vi "GUI.vi"() -> ()   [LabVIEW 2021]
uses:
  controls/UI Data.ctl
  controls/Data.ctl
  <vilib>/Utility/miscctls.llb/LVTextColorsTypeDef.ctl
  <vilib>/Instr/_visa.llb/VISA Flush IO Buffer Mask.ctl
  <vilib>/Instr/_visa.llb/VISA Set IO Buffer Mask.ctl
  2235c835-d075-488e-97a8-ff40b99ec252.vi
  7fd0a03c-babe-4245-89f2-70f68a4e02e0.vi
  1471845a-d6a4-4e2a-9e95-cd8e6e7553b6.vi
  855ea0af-0154-4148-8bb7-d6a0285b6b06.vi
  67ce05d8-96ad-4a67-b405-b48edab3017d.vi
  0a54dc2d-becf-406e-8766-49dcf30bcf8a.vi
  20f714a1-d882-48df-be09-57c36569b2f2.vi
  ebcdb7a2-2a2c-4ba1-9570-780fec90ea4c.vi
  d7b92f73-f523-4b2b-853d-7ace1ccfb4c3.vi
  5e66b44c-e304-46e7-babf-65c984714624.vi
  3f0796be-9eb5-410d-95a1-f686e7479b0e.vi
  a6c2df6f-6ad4-4eb4-a9bc-2f05b466e969.vi
  535851f3-05c5-415e-8a07-50860e4f08cf.vi
  3643a199-7bcb-4f24-a83d-5ca93d957abf.vi
  187f9bc3-0ed3-4701-b56c-3ff7ee860393.vi
  eb7b7dfd-645e-46e6-868f-ba0f7f713db4.vi
  <vilib>/ULx/Write.llb/ULx Write (Digital Bool 1Line 1Point).vi
  <vilib>/Instr/_visa.llb/VISA Configure Serial Port (Instr).vi
  <vilib>/ULx/Create Channel.llb/ULx Create Channel (DO-Digital Output).vi
  styles/colors.vi
  <vilib>/ULx/ULx_LV.dll
  <vilib>/NI/Progress Bar/Progress Bar.lvlib
  <vilib>/zip/NI_Unzip.lvlib
panel:
  in  "Stop button":bool
  in  "Run button":bool
  out "Status":string
  in  "Settings button":bool
  out "Console":string
  in  "Serial communication\n settings":T1={"COM"="", "baud rate"=115200, "data bits"=8, "parity"=enum."None", "stop bits"=10, "flow control"=enum."None", "delay"=50, "I/O channel"="", "Board IP"=""} {"stop bits" items=["1.0"=10, "1.5"=15, "2.0"=20]; "baud rate" max=921600; "data bits" max=16}
  in  "Paths":bool
  in  "Save button":bool
  out "version:":string
  in  "Path: 4.9.12.XXXX":path=path "C:/Users/ken_X/Documents/LabVIEW projects/Project-A/outset-medical/4.9.12.6034"
  in  "Path: Android OS":path=path "C:/Users/ken_X/Documents/LabVIEW projects/Project-A/outset-medical/Android OS"
  # "Serial communication\n settings"
  # "I/O Channel"
  # "Board IP"
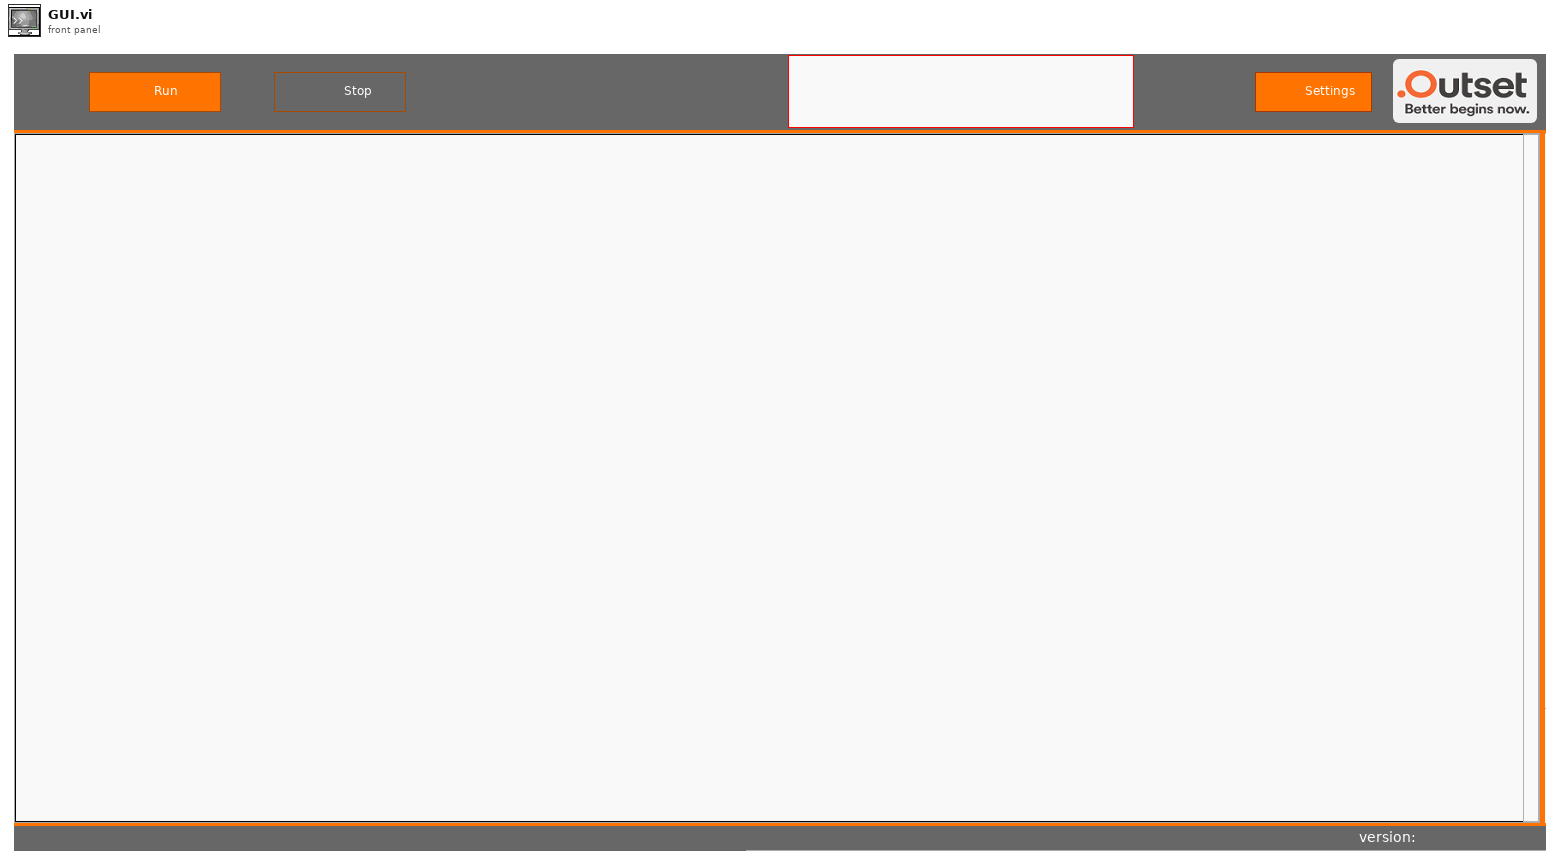
[diagram p1: front panel]
types:
  T1 = cluster{"COM":refnum<visa-resource-name>, "baud rate":u32, "data bits":u8, "parity":enum16{"None", "Odd", "Even", "Mark", "Space"}, "stop bits":u16, "flow control":enum16{"None", "XON/XOFF", "RTS/CTS", "DTR/DSR"}, "delay":u16, "I/O channel":refnum<k21>, "Board IP":string}
  T2 = typedef "Data.ctl" = cluster{"Console":refnum<vi>, "COM":refnum<visa-resource-name>, "Delay":u32, "IO task":refnum<k24>, "Python session":refnum<k35>, "Script path":path, "Media Url":string, "Media version":i32, "Attempts left":i32, "Version path":path, "Android path":path, "Python 2.7":path, "My temp":path, "Board IP":string, "ID Part":string, "Error":string, "Pass?":string}
  T3 = enum8{"Enabled", "Disabled", "Disabled and Grayed Out"}
  T4 = typedef "UI Data.ctl" = cluster{"settings splitter":refnum<vi>, "footer splitter":refnum<vi>, "Serial communication\n settings":refnum<vi>, "Path: Android OS":refnum<vi>, "Path: 4.9.12.XXXX":refnum<vi>}
  T5 = cluster{"primary color":u32, "secondary color":u32, "accent color":u32, "background color":u32, "accent s color":u32}
  T6 = cluster{"accent s color":u32, "accent s color":u32}
  T7 = cluster{"accent s color":u32, "accent color":u32}
  T8 = cluster{"primary color":u32, "primary color":u32}
  T9 = typedef "LVTextColorsTypeDef.ctl" = cluster{"Text Color":u32, "Background Color":u32}
  T10 = enum16{"open", "replace", "create", "open or create", "replace or create", "replace or create with confirmation"}
  T11 = cluster{"Android":path, "Version":path, "Labview Script":path, "Python 2.7":path, "My temp":path}
  T12 = typedef "VISA Set IO Buffer Mask.ctl" = u16
  T13 = typedef "VISA Flush IO Buffer Mask.ctl" = u16
  T14 = cluster{"secondary color":u32, "secondary color":u32}
  T15 = cluster{"Value":path, "Value":path, path, path, path}
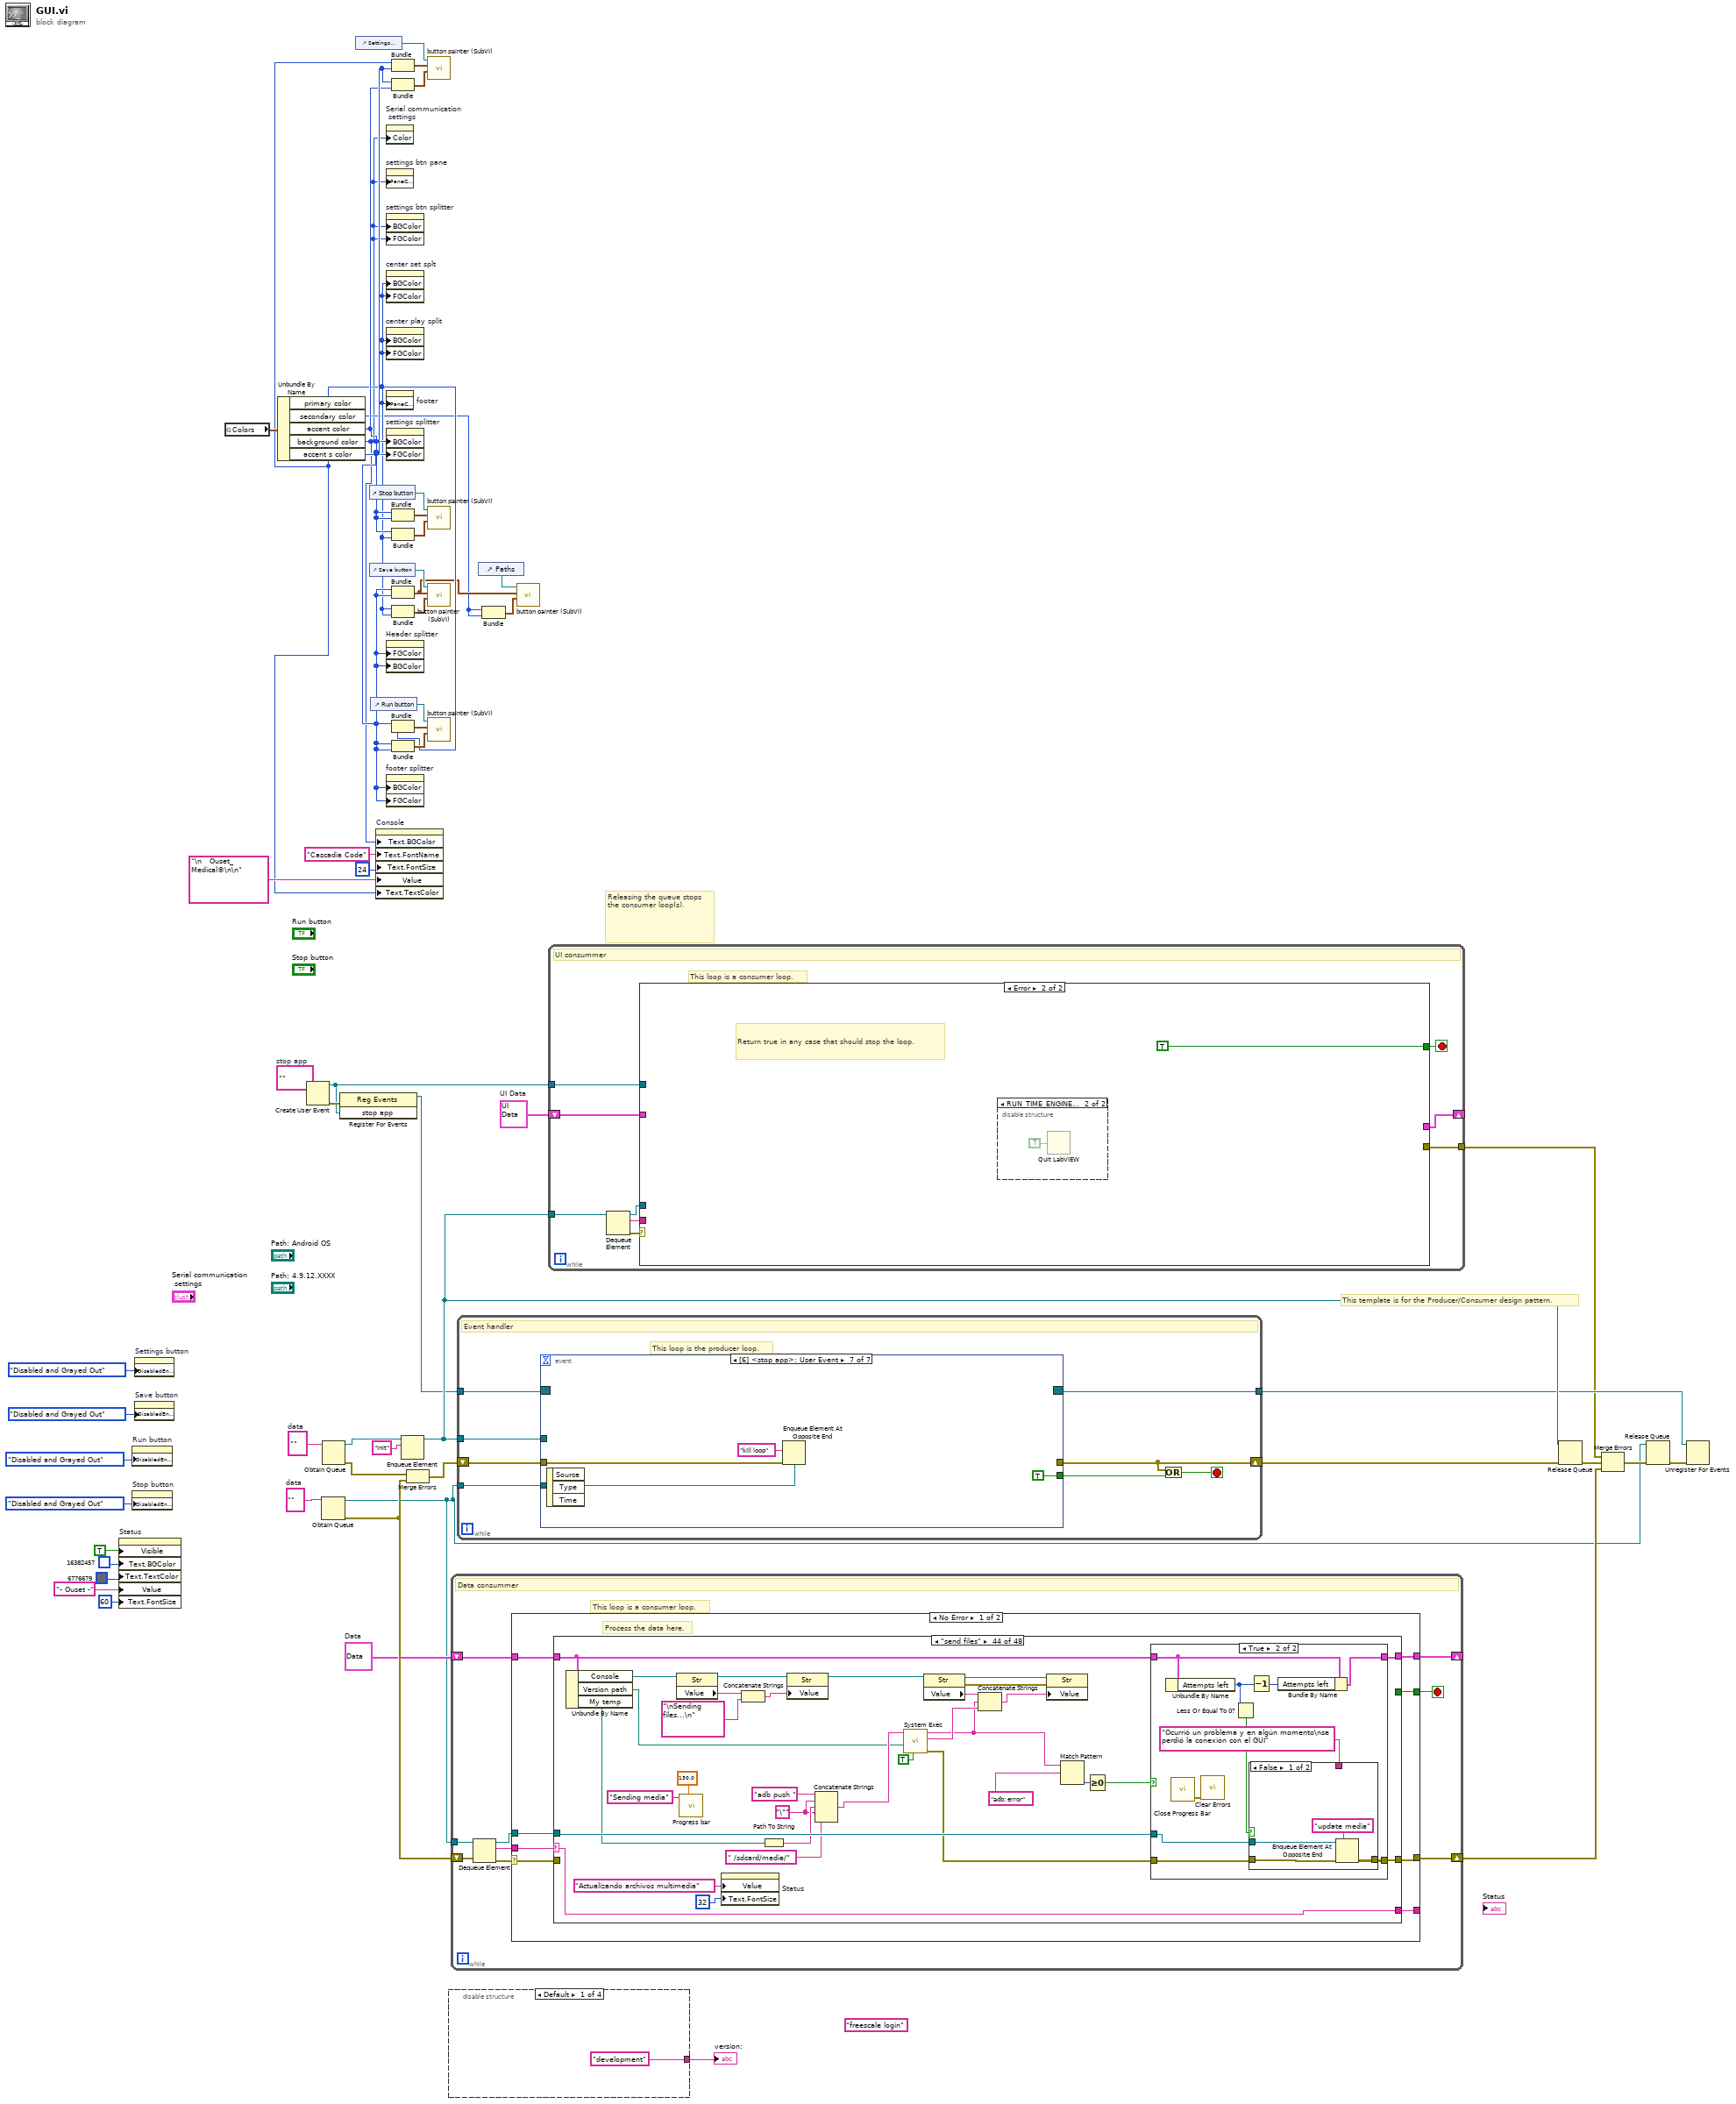
[diagram p0: block diagram]
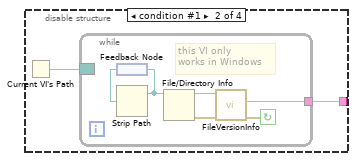
[diagram p2: hidden frame]
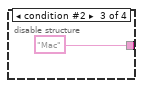
[diagram p3: hidden frame]
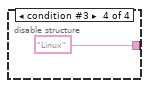
[diagram p4: hidden frame]
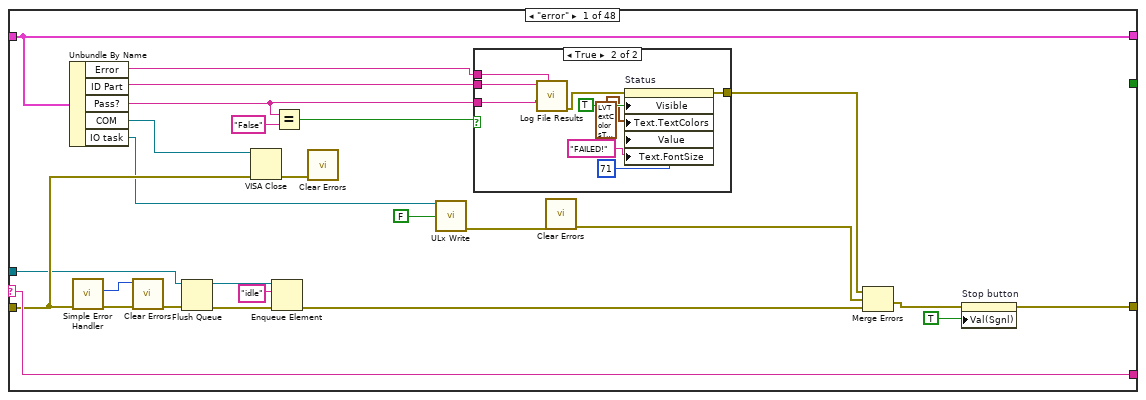
[diagram p5: hidden frame]
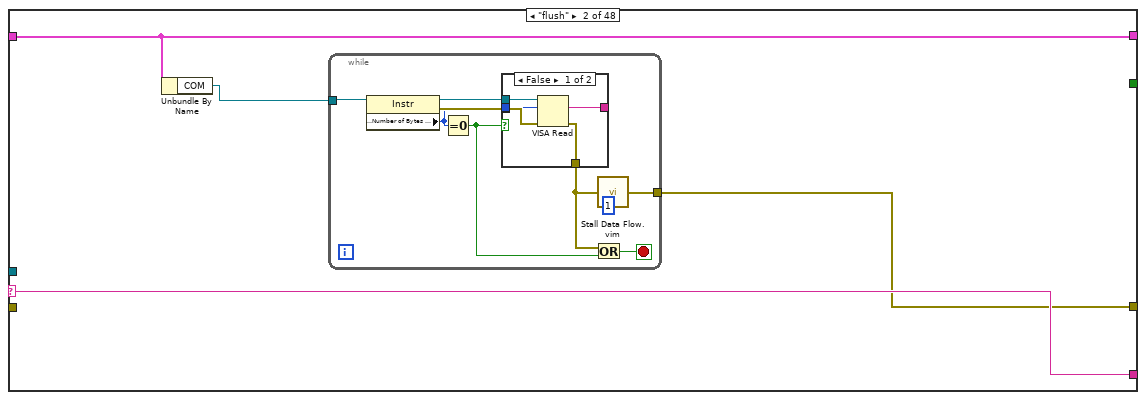
[diagram p7: hidden frame]
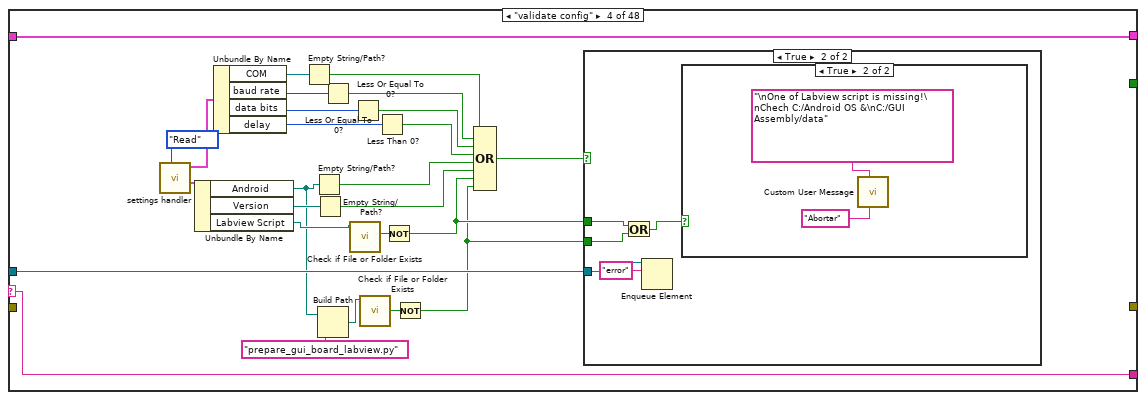
[diagram p10: hidden frame]
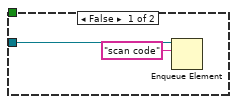
[diagram p11: hidden frame]
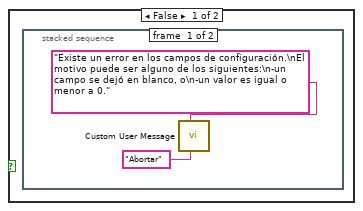
[diagram p12: hidden frame]
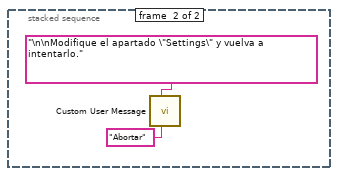
[diagram p13: hidden frame]
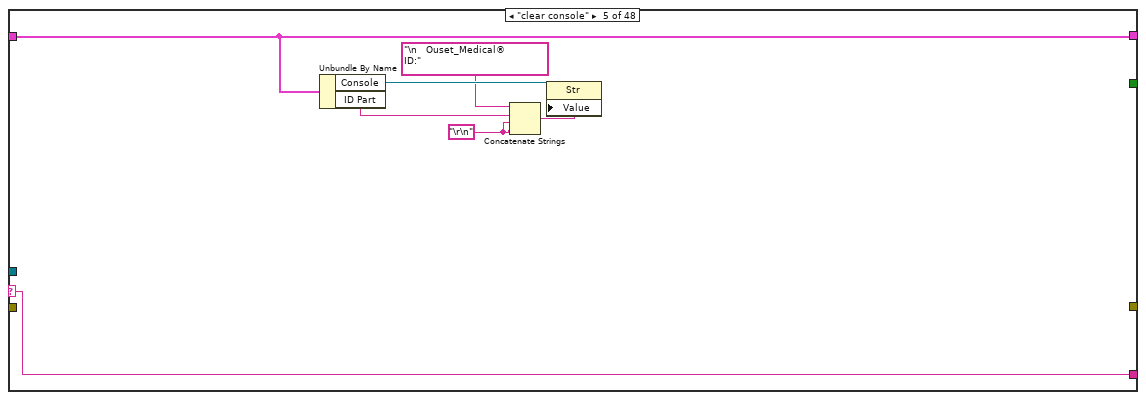
[diagram p14: hidden frame]
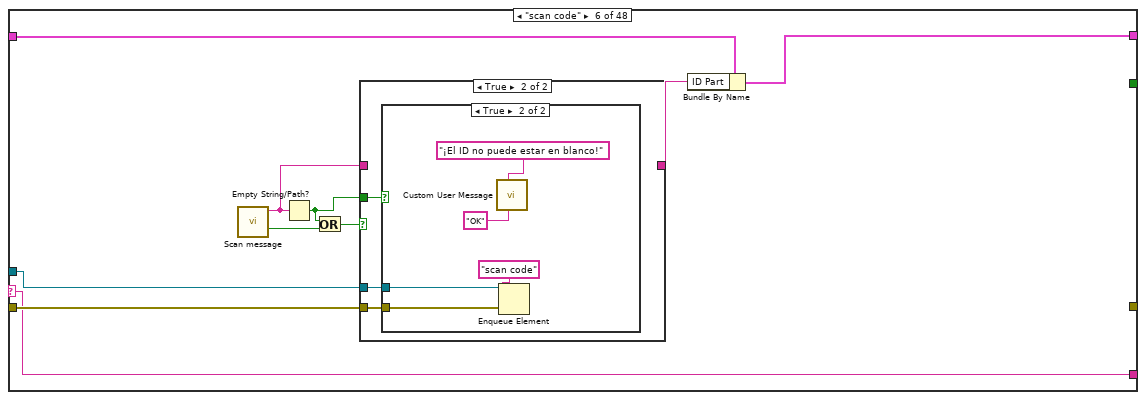
[diagram p15: hidden frame]
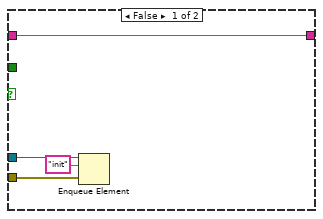
[diagram p16: hidden frame]
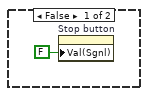
[diagram p17: hidden frame]
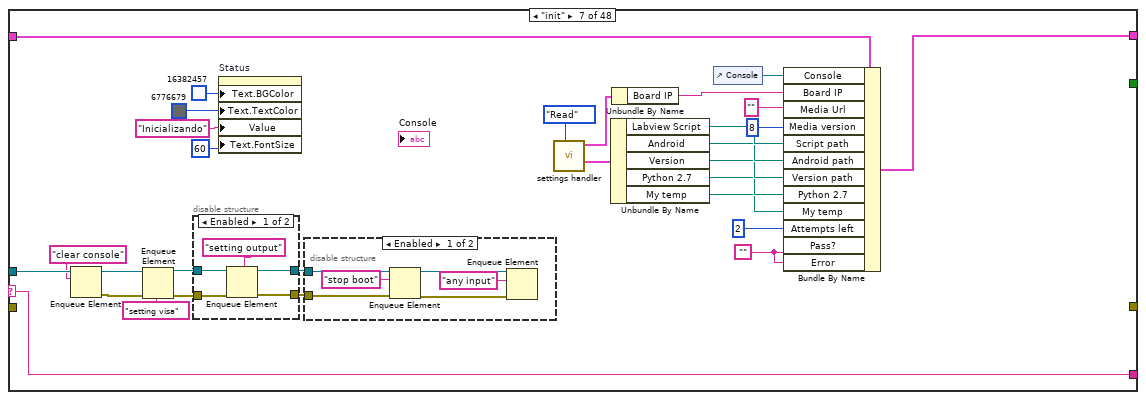
[diagram p18: hidden frame]
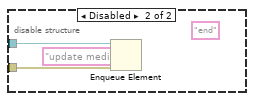
[diagram p20: hidden frame]
diagram:
  (unwired) "freescale login"
  w15 = T2 {"Console"=refnum, "COM"="", "Delay"=50, "IO task"=refnum, "Python session"=refnum, "Script path"=path "C:/Users/ken_X/Documents/LabVIEW projects/Project-A/Update_Media_bi.py", "Media Url"="", "Media version"=0, "Attempts left"=3, "Version path"=path "C:/Users/ken_X/Documents/LabVIEW projects/Project-A/Update_Media_bi.py", "Android path"=path "C:/Users/ken_X/Documents/LabVIEW projects/Project-A/Update_Media_bi.py", "Python 2.7"=path "C:/Users/ken_X/Documents/LabVIEW projects/Project-A/Update_Media_bi.py", "My temp"=path "C:/Users/ken_X/Documents/LabVIEW projects/Project-A/Update_Media_bi.py", "Board IP"="", "ID Part"="", "Error"="", "Pass?"=""}  # Data
  w33 = ""  # data
  w46 = ""  # stop app
  w50 = T4 {"settings splitter"=refnum, "footer splitter"=refnum, "Serial communication\n settings"=refnum, "Path: Android OS"=refnum, "Path: 4.9.12.XXXX"=refnum}  # UI Data
  w47 = ""  # data
  # "Releasing the queue stops the consumer loop(s)."
  # "This template is for the Producer/Consumer design pattern."
  n1 = property on="Status" class="Str"("Visible"=TRUE, "Text.BGColor"=u32 16382457 ("background color"), "Text.TextColor"=u32 6776679 ("primary color"), "Value"="- Ouset -" ("Status"), "Text.FontSize"=u32 60 ("Text.Font:Size")) -> ()  [unwired: 2 in, 2 out]
  n2 = property on="Run button" class="Bool (strict)"("DisabledEnum"=T3."Disabled and Grayed Out" ("Disabled")) -> ()  [unwired: 2 in, 2 out]
  n3 = property on="Stop button" class="Bool (strict)"("DisabledEnum"=T3."Disabled and Grayed Out" ("Disabled")) -> ()  [unwired: 2 in, 2 out]
  n4 = property on="Settings button" class="Bool (strict)"("DisabledEnum"=T3."Disabled and Grayed Out" ("Disabled")) -> ()  [unwired: 2 in, 2 out]
  n5 = property on="Save button" class="Bool (strict)"("DisabledEnum"=T3."Disabled and Grayed Out" ("Disabled")) -> ()  [unwired: 2 in, 2 out]
  n6 = global read "colors.vi" "Colors"() -> (w55:T5)
  n7 = Unbundle By Name(w55) -> ("primary color"=w22:u32, "secondary color"=w18:u32, "accent color"=w23:u32, "background color"=w16:u32, "accent s color"=w24:u32)
  n8 = Create User Event(user event datatype=w46) -> (user event=w44:refnum<user-event>, error out=w45:errorcluster)  [unwired: 1 in]
  n9 = Obtain Queue(element data type=w33) -> (queue out=w5:refnum<queue>, error out=w30:errorcluster)  [unwired: 4 in, 1 out]
  n10 = Obtain Queue(element data type=w47) -> (queue out=w53:refnum<queue>, error out=w32:errorcluster)  [unwired: 4 in, 1 out]
  n11 = register-events(error in=w45, w44) -> (reference out=w14:refnum<event-registration>)  [unwired: 1 in, 1 out]
  n12 = control-ref of="Settings button"() -> (w38:refnum<vi>)
  n13 = control-ref of="Stop button"() -> (w36:refnum<vi>)
  n14 = control-ref of="Save button"() -> (w37:refnum<vi>)
  n15 = control-ref of="Run button"() -> (w43:refnum<vi>)
  n16 = property on="Console" class="Str"("Text.BGColor"=w16, "Text.FontName"="Cascadia Code" ("Text.Font:Name"), "Text.FontSize"=u32 24 ("Text.Font:Size"), "Value"="\n   Ouset_Medical®\n\n" ("Console"), "Text.TextColor"=w24) -> ()  [unwired: 2 in, 2 out]
  n17 = property on="Serial communication\n settings" class="Clust (strict)"("Color"=w16) -> ()  [unwired: 2 in, 2 out]
  n18 = property on="settings btn pane" class="Pane"("PaneColor"=w16) -> ()  [unwired: 2 in, 2 out]
  n19 = property on="settings btn splitter" class="Splitter"("BGColor"=w16, "FGColor"=w16) -> ()  [unwired: 2 in, 2 out]
  n20 = property on="center set splt" class="Splitter"("BGColor"=w22, "FGColor"=w22) -> ()  [unwired: 2 in, 2 out]
  n21 = property on="center play split" class="Splitter"("BGColor"=w22, "FGColor"=w22) -> ()  [unwired: 2 in, 2 out]
  n22 = property on="footer" class="Pane"("PaneColor"=w22) -> ()  [unwired: 2 in, 2 out]
  n23 = property on="settings splitter" class="Splitter"("BGColor"=w23, "FGColor"=w23) -> ()  [unwired: 2 in, 2 out]
  n24 = property on="Header splitter" class="Splitter"("FGColor"=w23, "BGColor"=w23) -> ()  [unwired: 2 in, 2 out]
  n25 = property on="footer splitter" class="Splitter"("BGColor"=w23, "FGColor"=w23) -> ()  [unwired: 2 in, 2 out]
  n26 = Bundle("accent s color"=w24, "accent s color"=w24) -> (w40:T6)  [unwired: 1 in]
  n27 = Bundle("accent s color"=w24, "accent color"=w23) -> (w39:T7)  [unwired: 1 in]
  n28 = Bundle("accent color"=w23, "accent color"=w23) -> (w34:cluster{"accent color":u32, "accent color":u32})  [unwired: 1 in]
  n29 = Bundle("accent color"=w23, "primary color"=w22) -> (w35:cluster{"accent color":u32, "primary color":u32})  [unwired: 1 in]
  n30 = Bundle("accent color"=w23, "accent color"=w23) -> (w20:cluster{"accent color":u32, "accent color":u32})  [unwired: 1 in]
  n31 = Bundle("primary color"=w22, "primary color"=w22) -> (w19:T8)  [unwired: 1 in]
  n32 = Bundle("accent color"=w23, "primary color"=w22) -> (w41:cluster{"accent color":u32, "primary color":u32})  [unwired: 1 in]
  n33 = Bundle("accent color"=w23, "accent color"=w23) -> (w42:cluster{"accent color":u32, "accent color":u32})  [unwired: 1 in]
  n34 = Enqueue Element(queue=w53, element="init") -> (queue out=w52:refnum<queue>)  [unwired: 2 in, 2 out]
  n35 = Merge Errors(w32, w30) -> (w31:errorcluster)
  n36 = call "button painter (SubVI).vi"("Off state"=w39, "On state"=w40, "Button ref in"=w38) -> ()  [unwired: 9 in]
  n37 = call "button painter (SubVI).vi"("Off state"=w35, "On state"=w34, "Button ref in"=w36) -> ()  [unwired: 9 in]
  n38 = call "button painter (SubVI).vi"("Off state"=w19, "On state"=w20, "Button ref in"=w37) -> ()  [unwired: 9 in]
  n39 = call "button painter (SubVI).vi"("Off state"=w42, "On state"=w41, "Button ref in"=w43) -> ()  [unwired: 9 in]
  n40 = disable-structure "Conditional Disable Structure" shown="Default" {
    disable-tunnel: ["development" w57 "Mac" "Linux"] -> w13
    frame condition #0 (active) {
    }
    frame condition #1 {
      n41 = Current VI's Path() -> (path=w58:path)
      n42 = while {
        border: w58 -> [_]
        tunnel: [w59] -> w57
        stop <- w63 continue-if-true
        # "this VI only \nworks in Windows"
        n43 = feedback #1() -> (w62:path)
        n44 = Strip Path(path=w62) -> (stripped path=w61:path)  [unwired: 1 out]
        n45 = feedback-in #1(w61) -> ()
        n46 = File/Directory Info(path=w61) -> (path out=w60:path, error out=w64:errorcluster)  [unwired: 1 in, 5 out]
        n47 = call <vilib>:"FileVersionInfo.vi"("error in (no error)"=w64, "Application Path in"=w60) -> ("error out"=w63:errorcluster, "File Version Info"=w59:string)  [unwired: 6 in, 2 out]
      }
    }
    frame condition #2 {
    }
    frame condition #3 {
    }
  }
  "version:" <- w13
  n48 = while {
    tunnel: w5 -> [w75]
    shift-right: [w69] -> _
    shift-left: w15 -> [w70]
    shift-right: [w67] -> w8
    shift-left: w30 -> [w71]
    stop <- w68 stop-if-true
    # "This loop is a consumer loop."
    # "Data consummer"
    n49 = Dequeue Element(queue=w75, error in (no error)=w71) -> (queue out=w72:refnum<queue>, element=w73:string, error out=w74:errorcluster)  [unwired: 1 in, 1 out]
    n50 = case shown="No Error" w74 {
      selector: w74 -> [w78 w1835]
      tunnel: w73 -> [w83 _]
      tunnel: w72 -> [w82 w1843]
      tunnel: w70 -> [w81 w1842]
      tunnel: [w80 w1842] -> w69
      tunnel: [w79 "ERROR"] -> _
      tunnel: [w77 w1838] -> w67
      tunnel: [w76 _] -> w68
      frame No Error {
        # "Process the data here."
        n51 = case shown="\"send files\"" w83 {
          selector: w83 -> [w108 w121 w138 w148 w183 w187 w234 w264 w315 w363 w399 w441 w507 w541 w574 w638 w668 w707 w738 w801 w862 w903 w929 w989 w1032 w1054 w1091 w1126 w1179 w1217 w1268 w1291 w1345 w1363 w1385 w1425 w1469 w1505 w1530 w1553 w1591 w1629 w1662 w1708 w1759 w1779 w1788 w1804]
          tunnel: w82 -> [w97 _ _ w149 _ w194 w238 _ _ w364 w400 w444 w508 w545 w577 _ w669 w706 w739 w804 w852 _ w936 w990 _ w1056 w1093 w1128 w1180 w1219 _ w1293 w1347 _ w1380 w1418 w1463 w1507 w1527 w1556 w1594 w1632 w1655 w1710 w1761 _ _ w1800]
          tunnel: w81 -> [w86 w122 w139 w165 w185 w191 w237 w256 w321 w361 w413 w436 w490 w542 w569 w637 w666 w709 w736 w800 w836 w917 w922 w987 w1035 w1044 w1086 w1109 w1172 w1203 w1258 w1278 w1321 w1359 w1376 w1417 w1452 w1503 w1532 w1541 w1579 w1617 w1666 w1685 w1752 w1777 w1789 w1799]
          tunnel: [w86 w122 w139 w165 w185 w190 w235 w270 w325 w361 w413 w435 w489 w542 w570 w637 w666 w709 w736 w800 w835 w917 w921 w987 w1034 w1043 w1085 w1108 w1171 w1202 w1258 w1277 w1321 w1359 w1374 w1417 w1450 w1503 w1532 w1540 w1578 w1616 w1666 w1684 w1752 w1777 w1789 w1799] -> w80
          tunnel: [w108 w121 w138 w148 w183 w187 w234 w264 w315 w363 w399 w441 w507 w541 w574 w638 w668 w707 w738 w801 w862 w903 w929 w989 w1032 w1054 w1091 w1126 w1179 w1217 w1268 w1291 w1345 w1363 w1385 w1425 w1469 w1505 w1530 w1553 w1591 w1629 w1662 w1708 w1759 w1779 w1788 w1804] -> w79
          tunnel: w78 -> [w100 _ _ _ _ w195 _ _ w337 _ w404 _ _ _ _ _ _ _ _ w810 w850 _ w934 _ _ w1051 _ w1124 w1177 w1212 _ _ _ w1361 w1382 w1421 _ w1506 w1529 _ _ _ w1654 _ _ _ _ _]
          tunnel: [w103 w119 _ _ _ _ _ w262 w322 w358 w401 w437 w495 w540 w572 w629 w663 w704 w733 w803 w848 _ w933 w984 w1031 w1052 w1092 w1125 w1178 w1213 w1259 w1289 w1333 w1360 w1379 w1419 w1464 w1504 w1528 w1551 w1589 w1627 w1664 w1706 w1757 w1772 _ w1801] -> w77
          tunnel: [_ _ _ _ _ _ _ _ _ _ _ _ _ _ _ _ _ _ _ _ _ _ _ _ _ _ _ _ _ _ _ _ _ _ _ _ _ _ _ _ _ _ _ _ _ _ TRUE _] -> w76
          frame "error" {
            n52 = Unbundle By Name(w86) -> ("Error"=w92:string, "ID Part"=w93:string, "Pass?"=w94:string, "COM"=w105:refnum<visa-resource-name>, "IO task"=w91:refnum<k24>)
            n53 = call <vilib>:"Simple Error Handler.vi"("error in (no error)"=w100) -> ("code out"=w101:i32, "error out"=w98:errorcluster)  [unwired: 4 in, 3 out]
            n54 = call <vilib>:"Clear Errors.vi"("error in (no error)"=w98, "specific error code to clear (0: all)"=w101) -> ("error out"=w99:errorcluster)  [unwired: 4 in, 1 out]
            n55 = Flush Queue(queue=w97, error in (no error)=w99) -> (queue out=w107:refnum<queue>, error out=w106:errorcluster)  [unwired: 1 out]
            n56 = VISA Close(VISA resource name=w105, error in (no error)=w100) -> (error out=w102:errorcluster)
            n57 = Enqueue Element(queue=w107, element="idle", error in (no error)=w106) -> (error out=w88:errorcluster)  [unwired: 1 in, 2 out]
            n58 = Equal?(x=w94, y="False") -> (x = y?=w96:bool)
            n59 = call <vilib>:"Clear Errors.vi"("error in (no error)"=w102) -> ()  [unwired: 5 in, 2 out]
            n60 = call-poly <vilib>:"ULx Write.vi"("task in"=w91, "data"=FALSE) -> ("error out"=w85:errorcluster)  [unwired: 11 in, 2 out]
            n61 = case shown="True" w96 {
              tunnel: w93 -> [_ w118]
              tunnel: w94 -> [_ w117]
              tunnel: w92 -> [_ w116]
              tunnel: [_ w111] -> w89
              frame False {
              }
              frame True {
                n62 = call "Log File Results.vi"("Error"=w116, "Pass?"=w117, "Part Number"=w118) -> ("error out"=w112:errorcluster)  [unwired: 8 in]
                n63 = property on="Status" class="Str"(error in=w112, "Visible"=TRUE, "Text.TextColors"=T9 {"Text Color"=16777225, "Background Color"=16711680} ("Text.Text Colors"), "Value"="FAILED!" ("Status"), "Text.FontSize"=u32 71 ("Text.Font:Size")) -> (error out=w111:errorcluster)  [unwired: 1 in, 1 out]
              }
            }
            n64 = call <vilib>:"Clear Errors.vi"("error in (no error)"=w85) -> ("error out"=w84:errorcluster)  [unwired: 5 in, 1 out]
            n65 = Merge Errors(w89, w84, w88) -> (w87:errorcluster)
            n66 = property on="Stop button" class="Bool (strict)"(error in=w87, "Val(Sgnl)"=TRUE ("Value (Signaling)")) -> (error out=w103:errorcluster)  [unwired: 1 in, 1 out]
          }
          frame "flush" {
            n67 = Unbundle By Name(w122) -> ("COM"=w120:refnum<visa-resource-name>)
            n68 = while {
              tunnel: w120 -> [w131]
              tunnel: [w124] -> w119
              stop <- w129 stop-if-true
              n69 = property class="Instr"(reference=w131) -> (reference out=w130:refnum<visa-resource-name>, error out=w128:errorcluster, "Serial Settings:Number of Bytes at Serial Port"=w126:u32)  [unwired: 1 in]
              n70 = Equal To 0?(x=w126) -> (x = 0?=w127:bool)
              n71 = case shown="False" w127 {
                tunnel: w130 -> [w136 _]
                tunnel: w128 -> [w135 w137]
                tunnel: [w134 w137] -> w125
                tunnel: w126 -> [w133 _]
                tunnel: [w132 _] -> _
                frame False {
                  n72 = VISA Read(VISA resource name=w136, byte count=w133, error in (no error)=w135) -> (read buffer=w132:string, error out=w134:errorcluster)  [unwired: 2 out]
                }
                frame True {
                }
              }
              n73 = Or(x=w125, y=w127) -> (x .or. y?=w129:bool)
              n74 = call "Stall Data Flow.vim"("value in"=w125, "milliseconds to wait"=u32 1) -> ("value out"=w124:errorcluster)  [unwired: 1 out]
            }
          }
          frame "idle", Default {
          }
          frame "validate config" {
            n75 = call "settings handler.vi"("Operation"=enum16{"Open", "Write", "Read", "Close"}."Read") -> ("Paths read"=w163:T11, "Read"=w159:T1)  [unwired: 8 in, 1 out]
            n76 = Unbundle By Name(w163) -> ("Android"=w143:path, "Version"=w162:path, "Labview Script"=w147:path)
            n77 = Unbundle By Name(w159) -> ("COM"=w158:refnum<visa-resource-name>, "baud rate"=w157:u32, "data bits"=w156:u8, "delay"=w155:u16)
            n78 = Empty String/Path?(string/path=w158) -> (empty?=w151:bool)
            n79 = Empty String/Path?(string/path=w143) -> (empty?=w160:bool)
            n80 = Empty String/Path?(string/path=w162) -> (empty?=w161:bool)
            n81 = Build Path(base path=w143, name or relative path="prepare_gui_board_labview.py") -> (appended path=w144:path)
            n82 = Less Or Equal To 0?(x=w157) -> (x <= 0?=w152:bool)
            n83 = call <vilib>:"Check if File or Folder Exists.vi"("path"=w147) -> ("file or folder exists?"=w146:bool)  [unwired: 8 in, 2 out]
            n84 = Less Or Equal To 0?(x=w156) -> (x <= 0?=w153:bool)
            n85 = call <vilib>:"Check if File or Folder Exists.vi"("path"=w144) -> ("file or folder exists?"=w141:bool)  [unwired: 8 in, 2 out]
            n86 = Less Than 0?(x=w155) -> (x < 0?=w154:bool)
            n87 = Not(x=w146) -> (.not. x?=w145:bool)
            n88 = Not(x=w141) -> (.not. x?=w140:bool)
            n89 = Compound Arithmetic op=OR(w151, w152, w153, w154, w160, w161, w145, w140) -> (w150:bool)
            n90 = case shown="True" w150 {
              tunnel: w149 -> [w167 w172]
              tunnel: w145 -> [_ w170]
              tunnel: w140 -> [_ w169]
              frame False {
                n91 = Enqueue Element(queue=w167, element="scan code") -> ()  [unwired: 2 in, 3 out]
              }
              frame True {
                n92 = Or(x=w170, y=w169) -> (x .or. y?=w168:bool)
                n93 = Enqueue Element(queue=w172, element="error") -> ()  [unwired: 2 in, 3 out]
                n94 = case shown="True" w168 {
                  frame False {
                    n95 = stacked-sequence {
                      frame #0 {
                        n96 = call "Custom User Message.vi"("Button text (\"OK\")"="Abortar" ("Button text (\"OK\")"), "MSG"="Existe un error en los campos de configuración.\nEl motivo puede ser alguno de los siguientes:\n-un campo se dejó en blanco, o\n-un valor es igual o menor a 0." ("message")) -> ()  [unwired: 9 in, 1 out]
                      }
                      frame #1 {
                        n97 = call "Custom User Message.vi"("Button text (\"OK\")"="Abortar" ("Button text (\"OK\")"), "MSG"="\n\nModifique el apartado \"Settings\" y vuelva a intentarlo.") -> ()  [unwired: 9 in, 1 out]
                      }
                    }
                  }
                  frame True {
                    n98 = call "Custom User Message.vi"("Button text (\"OK\")"="Abortar" ("Button text (\"OK\")"), "MSG"="\nOne of Labview script is missing!\nChech C:/Android OS &\nC:/GUI Assembly/data" ("message")) -> ()  [unwired: 9 in, 1 out]
                  }
                }
              }
            }
          }
          frame "clear console" {
            w179 = "\r\n"
            n99 = Unbundle By Name(w185) -> ("Console"=w184:refnum<vi>, "ID Part"=w180:string)
            n100 = Concatenate Strings("\n   Ouset_Medical®         ID:" ("Value"), w180, w179, w179) -> (w182:string)
            n101 = property class="Str"(reference=w184, "Value"=w182) -> ()  [unwired: 1 in, 2 out]
          }
          frame "scan code" {
            n102 = call "Scan message.vi"() -> ("Abort?"=w193:bool, "out"=w188:string)  [unwired: 10 in]
            n103 = Empty String/Path?(string/path=w188) -> (empty?=w186:bool)
            n104 = Or(x=w186, y=w193) -> (x .or. y?=w192:bool)
            n105 = case shown="True" w192 {
              tunnel: w195 -> [w199 w200]
              tunnel: w194 -> [w198 w201]
              tunnel: [w196 _] -> w189
              tunnel: w188 -> [w196 _]
              tunnel: w186 -> [_ w202]
              frame False {
                n106 = Enqueue Element(queue=w198, element="init", error in (no error)=w199) -> ()  [unwired: 1 in, 3 out]
              }
              frame True {
                n107 = case shown="True" w202 {
                  tunnel: w201 -> [_ w207]
                  tunnel: w200 -> [_ w206]
                  frame False {
                    n108 = property on="Stop button" class="Bool (strict)"("Val(Sgnl)"=FALSE ("Value (Signaling)")) -> ()  [unwired: 2 in, 2 out]
                  }
                  frame True {
                    n109 = call "Custom User Message.vi"("Button text (\"OK\")"="OK" ("Button text (\"OK\")"), "MSG"="¡El ID no puede estar en blanco!") -> ()  [unwired: 9 in, 1 out]
                    n110 = Enqueue Element(queue=w207, element="scan code", error in (no error)=w206) -> ()  [unwired: 1 in, 3 out]
                  }
                }
              }
            }
            n111 = Bundle By Name(cluster=w191, "ID Part"=w189) -> (w190:T2)
          }
          frame "init" {
            w218 = ""
            n112 = Enqueue Element(queue=w238, element="clear console") -> (queue out=w221:refnum<queue>, error out=w222:errorcluster)  [unwired: 2 in, 1 out]
            n113 = Enqueue Element(queue=w221, element="setting visa", error in (no error)=w222) -> (queue out=w215:refnum<queue>, error out=w216:errorcluster)  [unwired: 1 in, 1 out]
            n114 = disable-structure shown="Enabled" {
              disable-tunnel: w216 -> [w243 w244]
              disable-tunnel: w215 -> [w242 w245]
              disable-tunnel: [w241 w245] -> w214
              disable-tunnel: [w240 w244] -> w213
              frame Enabled {
                n115 = Enqueue Element(queue=w242, element="setting output", error in (no error)=w243) -> (queue out=w241:refnum<queue>, error out=w240:errorcluster)  [unwired: 1 in, 1 out]
              }
              frame Disabled {
              }
            }
            n116 = property on="Status" class="Str"("Text.BGColor"=u32 16382457 ("background color"), "Text.TextColor"=u32 6776679 ("primary color"), "Value"="Inicializando" ("Status"), "Text.FontSize"=u32 60 ("Text.Font:Size")) -> ()  [unwired: 2 in, 2 out]
            n117 = disable-structure shown="Enabled" {
              disable-tunnel: w214 -> [w251 w254]
              disable-tunnel: w213 -> [w247 w252]
              frame Enabled {
                n118 = Enqueue Element(queue=w251, element="stop boot", error in (no error)=w247) -> (queue out=w249:refnum<queue>, error out=w248:errorcluster)  [unwired: 1 in, 1 out]
                n119 = Enqueue Element(queue=w249, element="any input", error in (no error)=w248) -> ()  [unwired: 1 in, 3 out]
              }
              frame Disabled {
                (unwired) "end" ("element")
                n120 = Enqueue Element(queue=w254, element="update media", error in (no error)=w252) -> ()  [unwired: 1 in, 3 out]
              }
            }
            n121 = call "settings handler.vi"("Operation"=enum16{"Open", "Write", "Read", "Close"}."Read") -> ("Paths read"=w229:T11, "Read"=w219:T1)  [unwired: 8 in, 1 out]
            n122 = Unbundle By Name(w229) -> ("Labview Script"=w228:path, "Android"=w226:path, "Version"=w225:path, "Python 2.7"=w224:path, "My temp"=w223:path)
            n123 = Unbundle By Name(w219) -> ("Board IP"=w220:string)
            n124 = control-ref of="Console"() -> (w236:refnum<vi>)
            n125 = Bundle By Name(cluster=w237, "Console"=w236, "Board IP"=w220, "Media Url"="", "Media version"=8, "Script path"=w228, "Android path"=w226, "Version path"=w225, "Python 2.7"=w224, "My temp"=w223, "Attempts left"=2, "Pass?"=w218, "Error"=w218) -> (w235:T2)
          }
          frame "setting visa" {
            n126 = call "settings handler.vi"("Operation"=enum16{"Open", "Write", "Read", "Close"}."Read") -> ("Read"=w275:T1)  [unwired: 8 in, 2 out]
            n127 = Unbundle By Name(w256) -> ("Console"=w261:refnum<vi>)
            n128 = Unbundle By Name(w275) -> ("COM"=w274:refnum<visa-resource-name>, "baud rate"=w273:u32, "data bits"=w272:u8, "parity"=w271:enum16{"None", "Odd", "Even", "Mark", "Space"}, "stop bits"=w268:u16, "flow control"=w269:enum16{"None", "XON/XOFF", "RTS/CTS", "DTR/DSR"}, "delay"=w267:u16)
            n129 = property class="Str"(reference=w261) -> (reference out=w260:refnum<vi>, "Value"=w259:string)  [unwired: 1 in, 1 out]
            n130 = Concatenate Strings(w259, ">setting VISA..." ("string")) -> (w258:string)
            n131 = property class="Str"(reference=w260, "Value"=w258) -> (reference out=w255:refnum<vi>)  [unwired: 1 in, 1 out]
            n132 = call-poly "VISA Configure Serial Port"("VISA resource name"=w274, "baud rate (9600)"=w273, "data bits (8)"=w272, "parity (0:none)"=w271, "stop bits (10: 1 bit)"=w268, "flow control (0:none)"=w269) -> ("VISA resource name out"=w266:refnum<visa-resource-name>, "error out"=w265:errorcluster)  [unwired: 4 in, 4 out]
            n133 = case shown="Error .." w265 {
              selector: w265 -> [w294 w306]
              tunnel: w266 -> [w296 w311]
              tunnel: [w288 w305] -> w262
              tunnel: [w297 _] -> w263
              tunnel: w255 -> [w284 _]
              frame No Error {
                w281 = T12 16 items=["I/O Receive Buffer"=16, "I/O Transmit Buffer"=32, "I/O Receive and Transmit Buffer"=48] ("Mask")
                w291 = T13 64 items=["Flush Receive Buffer"=16, "Write Transmit Buffer to Device"=32, "Flush Receive Buffer (No I/O)"=64, "Flush Transmit Buffer"=128] ("Mask")
                w295 = T13 128 items=["Flush Receive Buffer"=16, "Write Transmit Buffer to Device"=32, "Flush Receive Buffer (No I/O)"=64, "Flush Transmit Buffer"=128] ("Mask")
                n134 = VISA Flush I/O Buffer(VISA resource name=w296, mask (16)=w295, error in (no error)=w294) -> (VISA resource name out=w293:refnum<visa-resource-name>, error out=w292:errorcluster)
                n135 = VISA Flush I/O Buffer(VISA resource name=w293, mask (16)=w291, error in (no error)=w292) -> (VISA resource name out=w290:refnum<visa-resource-name>, error out=w289:errorcluster)
                n136 = property class="Str"(reference=w284) -> (reference out=w283:refnum<vi>, "Value"=w287:string)  [unwired: 1 in, 1 out]
                n137 = VISA Clear(VISA resource name=w290, error in (no error)=w289) -> (VISA resource name out=w282:refnum<visa-resource-name>, error out=w279:errorcluster)
                n138 = Concatenate Strings(w287, "\nOK!" ("string")) -> (w286:string)
                n139 = VISA Set I/O Buffer Size(VISA resource name=w282, mask (16)=w281, size (4096)=u32 16384, error in (no error)=w279) -> (VISA resource name out=w277:refnum<visa-resource-name>, error out=w278:errorcluster)
                n140 = property class="Str"(reference=w283, "Value"=w286) -> ()  [unwired: 1 in, 2 out]
                n141 = property class="Instr"(reference=w277, error in=w278, "General Settings:Timeout Value"=u32 5000) -> (reference out=w297:refnum<visa-resource-name>, error out=w288:errorcluster)
              }
              frame Error {
                w308 = T13 64 items=["Flush Receive Buffer"=16, "Write Transmit Buffer to Device"=32, "Flush Receive Buffer (No I/O)"=64, "Flush Transmit Buffer"=128] ("Mask")
                w309 = T13 128 items=["Flush Receive Buffer"=16, "Write Transmit Buffer to Device"=32, "Flush Receive Buffer (No I/O)"=64, "Flush Transmit Buffer"=128] ("Mask")
                n142 = VISA Flush I/O Buffer(VISA resource name=w311, mask (16)=w309, error in (no error)=w306) -> (VISA resource name out=w310:refnum<visa-resource-name>, error out=w307:errorcluster)
                n143 = VISA Flush I/O Buffer(VISA resource name=w310, mask (16)=w308, error in (no error)=w307) -> (VISA resource name out=w304:refnum<visa-resource-name>, error out=w303:errorcluster)
                n144 = VISA Clear(VISA resource name=w304, error in (no error)=w303) -> (VISA resource name out=w302:refnum<visa-resource-name>, error out=w301:errorcluster)
                n145 = VISA Close(VISA resource name=w302, error in (no error)=w301) -> (error out=w305:errorcluster)
                n146 = call "Custom User Message.vi"("Button text (\"OK\")"="OK" ("Button text (\"OK\")"), "MSG"="Existe un problema al conectarse por modo serial vía VISA.\nAsegúrese que todo esté bien configurado.") -> ()  [unwired: 9 in, 1 out]
              }
            }
            n147 = Bundle By Name(cluster=w256, "COM"=w263, "Delay"=w267) -> (w270:T2)
          }
          frame "setting output" {
            w340 = 1 items=["OneChannelForEachLine", "OneChannelForAllLines"] ("line grouping")
            n148 = call "settings handler.vi"("Operation"=enum16{"Open", "Write", "Read", "Close"}."Read") -> ("Read"=w335:T1)  [unwired: 8 in, 2 out]
            n149 = Unbundle By Name(w321) -> ("Console"=w320:refnum<vi>)
            n150 = Unbundle By Name(w335) -> ("I/O channel"=w334:refnum<k21>)
            n151 = property class="Str"(reference=w320) -> (reference out=w319:refnum<vi>, "Value"=w318:string)  [unwired: 1 in, 1 out]
            n152 = Concatenate Strings(w318, "\n>setting output..." ("string")) -> (w317:string)
            n153 = call-poly <vilib>:"ULx Create Virtual Channel.vi"("lines"=w334, "line grouping"=w340, "error in"=w337) -> ("task out"=w339:refnum<k24>, "error out"=w338:errorcluster)  [unwired: 11 in]
            n154 = call <vilib>:"ULx Start Task.vi"("task in"=w339, "error in"=w338) -> ("task out"=w327:refnum<k24>, "error out"=w326:errorcluster)  [unwired: 12 in]
            n155 = property class="Str"(reference=w319, "Value"=w317) -> (reference out=w314:refnum<vi>)  [unwired: 1 in, 1 out]
            n156 = call-poly <vilib>:"ULx Write.vi"("task in"=w327, "data"=FALSE, "error in"=w326) -> ("task out"=w328:refnum<k24>, "error out"=w331:errorcluster)  [unwired: 10 in, 1 out]
            n157 = property on="Status" class="Str"("Value"="Configurando la salida de voltaje" ("Status"), "Text.FontSize"=u32 34 ("Text.Font:Size")) -> ()  [unwired: 2 in, 2 out]
            n158 = call "Stall Data Flow.vim"("value in"=w331, "milliseconds to wait"=u32 4000) -> ("value out"=w329:errorcluster)  [unwired: 1 out]
            n159 = call-poly <vilib>:"ULx Write.vi"("task in"=w328, "data"=TRUE, "error in"=w329) -> ("task out"=w324:refnum<k24>, "error out"=w323:errorcluster)  [unwired: 10 in, 1 out]
            n160 = case shown="Error .." w323 {
              selector: w323 -> [w346 w347]
              tunnel: [w346 w347] -> w322
              tunnel: w314 -> [w342 _]
              frame No Error {
                n161 = property class="Str"(reference=w342) -> (reference out=w341:refnum<vi>, "Value"=w345:string)  [unwired: 1 in, 1 out]
                n162 = Concatenate Strings(w345, "\nOK!" ("string")) -> (w344:string)
                n163 = property class="Str"(reference=w341, "Value"=w344) -> ()  [unwired: 1 in, 2 out]
              }
              frame Error {
                n164 = call "Custom User Message.vi"("Button text (\"OK\")"="OK" ("Button text (\"OK\")"), "MSG"="\nExiste un problema al comunicarse con la DAQ.\nAsegúrese que el cable USB \nque sale del gabinete este conectado \ny funcionando.  \n") -> ()  [unwired: 9 in, 1 out]
              }
            }
            n165 = Bundle By Name(cluster=w321, "IO task"=w324) -> (w325:T2)
          }
          frame "stop boot" {
            n166 = Unbundle By Name(w361) -> ("Console"=w355:refnum<vi>, "COM"=w359:refnum<visa-resource-name>)
            n167 = property class="Str"(reference=w355) -> (reference out=w354:refnum<vi>, "Value"=w356:string)  [unwired: 1 in, 1 out]
            n168 = Concatenate Strings(w356, "\n>Waiting for response from the Serial Port" ("string")) -> (w357:string)
            n169 = property class="Str"(reference=w354, "Value"=w357) -> (reference out=w353:refnum<vi>)  [unwired: 1 in, 1 out]
            n170 = property on="Status" class="Str"("Value"="Deteniendo el proceso de inicio" ("Status"), "Text.FontSize"=u32 34 ("Text.Font:Size")) -> ()  [unwired: 2 in, 2 out]
            n171 = while {
              shift-right: [w388] -> _
              shift-left: w359 -> [w385]
              tunnel: [w366] -> w360
              tunnel: [w381] -> w362
              tunnel: w353 -> [w367]
              i -> [w376]
              stop <- w379 stop-if-true
              # "Serial Write and Read Loop"
              n172 = property class="Instr"(reference=w385) -> (reference out=w384:refnum<visa-resource-name>, error out=w383:errorcluster, "Serial Settings:Number of Bytes at Serial Port"=w382:u32)  [unwired: 1 in]
              n173 = property class="Str"(reference=w367) -> (reference out=w374:refnum<vi>, "Value"=w371:string)  [unwired: 1 in, 1 out]
              n174 = Equal To 0?(x=w376) -> (x = 0?=w375:bool)
              n175 = VISA Read(VISA resource name=w384, byte count=w382, error in (no error)=w383) -> (VISA resource name out=w388:refnum<visa-resource-name>, read buffer=w370:string, error out=w387:errorcluster)  [unwired: 1 out]
              n176 = Concatenate Strings(w371, w370) -> (w372:string)
              n177 = call "Elapsed stop"("Time Target (s)"=15.0, "Reset"=w375) -> ("Time has Elapsed"=w378:bool)  [unwired: 10 in, 7 out]
              n178 = call "Stall Data Flow.vim"("value in"=w387, "milliseconds to wait"=u32 1) -> ("value out"=w366:errorcluster)  [unwired: 1 out]
              n179 = property class="Str"(reference=w374, "Value"=w372) -> (reference out=w369:refnum<vi>)  [unwired: 1 in, 1 out]
              n180 = Match Pattern(string=w370, regular expression="Hit any key") -> (offset past match=w386:i32)  [unwired: 1 in, 3 out]
              n181 = Greater Or Equal To 0?(x=w386) -> (x >= 0?=w381:bool)
              n182 = property class="Str"(reference=w369, "Text.Scroll Position"=u32 4294967295) -> ()  [unwired: 1 in, 2 out]
              n183 = Or(x=w366, y=w381) -> (x .or. y?=w380:bool)
              n184 = Or(x=w380, y=w378) -> (x .or. y?=w379:bool)
            }
            n185 = case shown="True" w362 {
              tunnel: w364 -> [w394 w395]
              tunnel: w360 -> [w392 w397]
              tunnel: [w391 w396] -> w358
              frame False {
                n186 = Enqueue Element At Opposite End(queue=w394, element="error", error in (no error)=w392) -> (error out=w391:errorcluster)  [unwired: 1 in, 2 out]
                n187 = call "Custom User Message.vi"("Button text (\"OK\")"="OK" ("Button text (\"OK\")"), "MSG"="\nParece ser que del otro lado de la conexión \nno se encuentra el GUI. Revise el cable de\ncomunicación serial") -> ()  [unwired: 9 in, 1 out]
              }
              frame True {
                n188 = Enqueue Element(queue=w395, element="clear console", error in (no error)=w397) -> (error out=w396:errorcluster)  [unwired: 1 in, 2 out]
              }
            }
          }
          frame "any input" {
            w408 = "a" ("write buffer")
            n189 = Unbundle By Name(w413) -> ("Console"=w406:refnum<vi>, "COM"=w403:refnum<visa-resource-name>)
            n190 = property class="Str"(reference=w406) -> (reference out=w411:refnum<vi>, error out=w405:errorcluster, "Value"=w412:string)  [unwired: 1 in]
            n191 = VISA Write(VISA resource name=w403, write buffer=w408, error in (no error)=w404) -> (error out=w402:errorcluster)  [unwired: 2 out]
            n192 = Concatenate Strings(w412, ">" ("string"), w408, "\r") -> (w410:string)
            n193 = property class="Str"(reference=w411, error in=w405, "Value"=w410) -> ()  [unwired: 2 out]
            n194 = case shown="Error .." w402 {
              selector: w402 -> [w423 w429]
              tunnel: [w425 w427] -> w401
              tunnel: w400 -> [w421 w428]
              frame No Error {
                n195 = Enqueue Element At Opposite End(queue=w421, element="flush", error in (no error)=w423) -> (queue out=w420:refnum<queue>, error out=w422:errorcluster)  [unwired: 1 in, 1 out]
                n196 = Enqueue Element(queue=w420, element="delay", error in (no error)=w422) -> (queue out=w417:refnum<queue>, error out=w414:errorcluster)  [unwired: 1 in, 1 out]
                n197 = Enqueue Element(queue=w417, element="clear console", error in (no error)=w414) -> (queue out=w416:refnum<queue>, error out=w415:errorcluster)  [unwired: 1 in, 1 out]
                n198 = Enqueue Element(queue=w416, element="destroyenv", error in (no error)=w415) -> (error out=w425:errorcluster)  [unwired: 1 in, 2 out]
              }
              frame Error {
                n199 = Enqueue Element(queue=w428, element="init", error in (no error)=w429) -> (error out=w427:errorcluster)  [unwired: 1 in, 2 out]
              }
            }
          }
          frame "destroyenv" {
            n200 = Unbundle By Name(w436) -> ("Console"=w443:refnum<vi>, "COM"=w442:refnum<visa-resource-name>)  [unwired: 1 out]
            n201 = Concatenate Strings(w441, "\r") -> (w439:string)
            n202 = VISA Write(VISA resource name=w442, write buffer=w439) -> (VISA resource name out=w446:refnum<visa-resource-name>, error out=w438:errorcluster)  [unwired: 1 in, 1 out]
            n203 = property on="Status" class="Str"("Value"="Configurando las variables de entorno" ("Status"), "Text.FontSize"=u32 32 ("Text.Font:Size")) -> ()  [unwired: 2 in, 2 out]
            n204 = while {
              shift-right: [w487] -> w445
              shift-left: w446 -> [w482]
              tunnel: [w472] -> w433
              tunnel: w438 -> [w481]
              tunnel: w443 -> [w474]
              tunnel: [w465] -> w434
              i -> [w468]
              stop <- w466 stop-if-true
              # "Serial Write and Read Loop"
              n205 = property class="Str"(reference=w474) -> (reference out=w477:refnum<vi>, "Value"=w473:string)  [unwired: 1 in, 1 out]
              n206 = property class="Instr"(reference=w482, error in=w481) -> (reference out=w480:refnum<visa-resource-name>, error out=w479:errorcluster, "Serial Settings:Number of Bytes at Serial Port"=w478:u32)
              n207 = Equal To 0?(x=w468) -> (x = 0?=w469:bool)
              n208 = VISA Read(VISA resource name=w480, byte count=w478, error in (no error)=w479) -> (VISA resource name out=w487:refnum<visa-resource-name>, read buffer=w475:string, error out=w486:errorcluster)  [unwired: 1 out]
              n209 = call "Elapsed stop2"("Time Target (s)"=10.0, "Reset"=w469) -> ("Time has Elapsed"=w465:bool)  [unwired: 10 in, 7 out]
              n210 = call "Stall Data Flow.vim"("value in"=w486, "milliseconds to wait"=u32 5) -> ("value out"=w472:errorcluster)  [unwired: 1 out]
              n211 = Concatenate Strings(w473, w475) -> (w476:string)
              n212 = Match Pattern(string=w475, regular expression="done") -> (offset past match=w484:i32)  [unwired: 1 in, 3 out]
              n213 = Greater Or Equal To 0?(x=w484) -> (x >= 0?=w483:bool)
              n214 = property class="Str"(reference=w477, "Value"=w476) -> ()  [unwired: 1 in, 2 out]
              n215 = Or(x=w472, y=w483) -> (x .or. y?=w467:bool)
              n216 = Or(x=w467, y=w465) -> (x .or. y?=w466:bool)
            }
            n217 = case shown="False" w434 {
              tunnel: w445 -> [_ _]
              tunnel: w444 -> [w451 w463]
              tunnel: [w449 w462] -> w437
              tunnel: w436 -> [w453 w461]
              tunnel: [w453 w460] -> w435
              tunnel: w433 -> [w447 w457]
              frame False {
                n218 = Enqueue Element(queue=w451, element="delay", error in (no error)=w447) -> (queue out=w448:refnum<queue>, error out=w450:errorcluster)  [unwired: 1 in, 1 out]
                n219 = Enqueue Element(queue=w448, element="send file", error in (no error)=w450) -> (error out=w449:errorcluster)  [unwired: 1 in, 2 out]
              }
              frame True {
                n220 = call "Custom User Message.vi"("Button text (\"OK\")"="Abortar" ("Button text (\"OK\")"), "MSG"="Parece ser que hubo un problema \nal mandar el comando \"destroyenv\"\n") -> ()  [unwired: 9 in, 1 out]
                n221 = Enqueue Element At Opposite End(queue=w463, element="error", error in (no error)=w457) -> (error out=w462:errorcluster)  [unwired: 1 in, 2 out]
                n222 = Bundle By Name(cluster=w461, "Error"="Error al destruir las\nvariables de entorno", "Pass?"="False") -> (w460:T2)
              }
            }
          }
          frame "send file" {
            n223 = Unbundle By Name(w490) -> ("Console"=w488:refnum<vi>, "COM"=w498:refnum<visa-resource-name>, "Android path"=w493:path)
            n224 = String To Path(string="gui_env.txt") -> (path=w492:path)
            n225 = Build Path(base path=w493, name or relative path=w492) -> (appended path=w491:path)
            n226 = Open/Create/Replace File(file path (use dialog)=w491, operation (0:open)=T10."open") -> (refnum out=w506:refnum<file>, error out=w504:errorcluster)  [unwired: 4 in, 1 out]
            n227 = Read from Text File(file (use dialog)=w506, error in=w504) -> (text=w502:string, error out=w496:errorcluster)  [unwired: 2 in, 2 out]
            n228 = Spreadsheet String To Array(delimiter (Tab)="\n", format string="%s", spreadsheet string=w502, array type (2D Dbl)=string[] []) -> (array=w499:string[])
            n229 = for {
              tunnel: w499 -> [w524] mode=indexing
              tunnel: w498 -> [w526]
              shift-right: [w516] -> w497
              shift-left: w496 -> [w525]
              tunnel: w488 -> [w512]
              stop <- w516 stop-if-true
              n230 = Concatenate Strings(w524, "\r") -> (w523:string)
              n231 = VISA Write(VISA resource name=w526, write buffer=w523, error in (no error)=w525) -> (VISA resource name out=w521:refnum<visa-resource-name>, error out=w519:errorcluster)  [unwired: 1 out]
              n232 = call "Stall Data Flow.vim"("value in"=w519, "milliseconds to wait"=u32 50) -> ("value out"=w510:errorcluster)  [unwired: 1 out]
              n233 = property class="Instr"(reference=w521, error in=w510) -> (reference out=w520:refnum<visa-resource-name>, error out=w518:errorcluster, "Serial Settings:Number of Bytes at Serial Port"=w517:u32)
              n234 = property class="Str"(reference=w512) -> (reference out=w515:refnum<vi>, "Value"=w514:string)  [unwired: 1 in, 1 out]
              n235 = VISA Read(VISA resource name=w520, byte count=w517, error in (no error)=w518) -> (read buffer=w511:string, error out=w516:errorcluster)  [unwired: 2 out]
              n236 = Concatenate Strings(w514, w511) -> (w513:string)
              n237 = property class="Str"(reference=w515, "Value"=w513) -> ()  [unwired: 1 in, 2 out]
            }
            n238 = case shown="No Error" w497 {
              selector: w497 -> [w529 w536]
              tunnel: w508 -> [w531 w538]
              tunnel: [w528 w536] -> w495
              tunnel: w490 -> [w527 w535]
              tunnel: [w527 w534] -> w489
              frame No Error {
                n239 = Enqueue Element(queue=w531, element="read buffer", error in (no error)=w529) -> (error out=w528:errorcluster)  [unwired: 1 in, 2 out]
              }
              frame Error {
                n240 = Enqueue Element At Opposite End(queue=w538, element="error") -> ()  [unwired: 2 in, 3 out]
                n241 = Bundle By Name(cluster=w535, "Error"="Error al mandar gui_env.txt", "Pass?"="False") -> (w534:T2)
              }
            }
          }
          frame "read buffer" {
            n242 = Unbundle By Name(w542) -> ("Console"=w539:refnum<vi>, "COM"=w543:refnum<visa-resource-name>)
            n243 = while {
              tunnel: [w548] -> w546
              tunnel: w543 -> [w554]
              tunnel: w539 -> [w549]
              stop <- w559 stop-if-true
              n244 = property class="Instr"(reference=w554) -> (reference out=w560:refnum<visa-resource-name>, error out=w558:errorcluster, "Serial Settings:Number of Bytes at Serial Port"=w556:u32)  [unwired: 1 in]
              n245 = Equal To 0?(x=w556) -> (x = 0?=w557:bool)
              n246 = case shown="False" w557 {
                tunnel: w560 -> [w565 _]
                tunnel: w558 -> [w564 w566]
                tunnel: [w563 w566] -> w555
                tunnel: w556 -> [w562 _]
                tunnel: [w561 _] -> w552
                frame False {
                  n247 = VISA Read(VISA resource name=w565, byte count=w562, error in (no error)=w564) -> (read buffer=w561:string, error out=w563:errorcluster)  [unwired: 2 out]
                }
                frame True {
                }
              }
              n248 = Or(x=w555, y=w557) -> (x .or. y?=w559:bool)
              n249 = call "Stall Data Flow.vim"("value in"=w555, "milliseconds to wait"=u32 5) -> ("value out"=w548:errorcluster)  [unwired: 1 out]
              n250 = property class="Str"(reference=w549) -> (reference out=w550:refnum<vi>, "Value"=w553:string)  [unwired: 1 in, 1 out]
              n251 = Concatenate Strings(w553, w552) -> (w551:string)
              n252 = property class="Str"(reference=w550, "Value"=w551) -> ()  [unwired: 1 in, 2 out]
            }
            n253 = Enqueue Element(queue=w545, element="saveenv", error in (no error)=w546) -> (error out=w540:errorcluster)  [unwired: 1 in, 2 out]
          }
          frame "saveenv" {
            n254 = Unbundle By Name(w569) -> ("Console"=w576:refnum<vi>, "COM"=w578:refnum<visa-resource-name>)  [unwired: 1 out]
            n255 = Concatenate Strings("\r", w574, "\r") -> (w575:string)
            n256 = VISA Write(VISA resource name=w578, write buffer=w575) -> (VISA resource name out=w581:refnum<visa-resource-name>, error out=w580:errorcluster)  [unwired: 1 in, 1 out]
            n257 = while {
              shift-right: [w626] -> w579
              shift-left: w581 -> [w621]
              tunnel: [w607] -> w567
              tunnel: w580 -> [w620]
              tunnel: w576 -> [w612]
              tunnel: [w608] -> w568
              stop <- w625 stop-if-true
              # "Serial Write and Read Loop"
              n258 = property class="Instr"(reference=w621, error in=w620) -> (reference out=w619:refnum<visa-resource-name>, error out=w618:errorcluster, "Serial Settings:Number of Bytes at Serial Port"=w617:u32)
              n259 = property class="Str"(reference=w612) -> (reference out=w616:refnum<vi>, "Value"=w614:string)  [unwired: 1 in, 1 out]
              n260 = VISA Read(VISA resource name=w619, byte count=w617, error in (no error)=w618) -> (VISA resource name out=w626:refnum<visa-resource-name>, read buffer=w613:string, error out=w624:errorcluster)  [unwired: 1 out]
              n261 = Concatenate Strings(w614, w613) -> (w615:string)
              n262 = call "Stall Data Flow.vim"("value in"=w624, "milliseconds to wait"=u32 5) -> ("value out"=w607:errorcluster)  [unwired: 1 out]
              n263 = Match Pattern(string=w613, regular expression="done") -> (offset past match=w622:i32)  [unwired: 1 in, 3 out]
              n264 = property class="Str"(reference=w616, "Value"=w615) -> (reference out=w611:refnum<vi>, error out=w609:errorcluster)  [unwired: 1 in]
              n265 = Greater Or Equal To 0?(x=w622) -> (x >= 0?=w608:bool)
              n266 = property class="Str"(reference=w611, error in=w609, "Text.Scroll Position"=u32 4294967295) -> ()  [unwired: 2 out]
              n267 = Or(x=w607, y=w608) -> (x .or. y?=w625:bool)
            }
            n268 = case shown="False" w568 {
              tunnel: w579 -> [_ _]
              tunnel: w577 -> [w590 w593]
              tunnel: [w589 w597] -> w572
              tunnel: [w588 w601] -> w570
              tunnel: w569 -> [w587 w601]
              tunnel: w567 -> [w584 w596]
              frame False {
                n269 = Enqueue Element At Opposite End(queue=w590, element="error", error in (no error)=w584) -> (error out=w589:errorcluster)  [unwired: 1 in, 2 out]
                n270 = call "Custom User Message.vi"("Button text (\"OK\")"="Abortar" ("Button text (\"OK\")"), "MSG"="Surgió un error al guardar \nlas variables de entorno") -> ()  [unwired: 9 in, 1 out]
                n271 = Bundle By Name(cluster=w587, "Error"="Error al salvar las variables de entorno", "Pass?"="False") -> (w588:T2)
              }
              frame True {
                n272 = Enqueue Element(queue=w593, element="flush", error in (no error)=w596) -> (queue out=w594:refnum<queue>, error out=w595:errorcluster)  [unwired: 1 in, 1 out]
                n273 = Enqueue Element(queue=w594, element="clear console", error in (no error)=w595) -> (queue out=w604:refnum<queue>, error out=w603:errorcluster)  [unwired: 1 in, 1 out]
                n274 = Enqueue Element(queue=w604, element="reboot", error in (no error)=w603) -> (queue out=w600:refnum<queue>, error out=w599:errorcluster)  [unwired: 1 in, 1 out]
                n275 = Enqueue Element(queue=w600, element="udp mode", error in (no error)=w599) -> (error out=w597:errorcluster)  [unwired: 1 in, 2 out]
              }
            }
          }
          frame "reboot" {
            n276 = Unbundle By Name(w637) -> ("Console"=w631:refnum<vi>, "IO task"=w636:refnum<k24>)
            n277 = property on="Status" class="Str"("Value"="Reiniciando" ("Status"), "Text.FontSize"=u32 60 ("Text.Font:Size")) -> ()  [unwired: 2 in, 2 out]
            n278 = disable-structure shown="Enabled" {
              disable-tunnel: w636 -> [w640 _]
              disable-tunnel: [w639 _] -> w629
              frame Enabled {
                n279 = flat-sequence {
                  tunnel: w640 -> [w648]
                  tunnel: [w646] -> w644
                  tunnel: [w645] -> w643
                  tunnel: w644 -> [w651]
                  tunnel: [w651] -> w642
                  tunnel: w643 -> [w649]
                  tunnel: [w649] -> w641
                  tunnel: w642 -> [w655]
                  tunnel: w641 -> [w653]
                  tunnel: [w652] -> w639
                  frame #0 {
                    # "turn off display"
                    n280 = call-poly <vilib>:"ULx Write.vi"("task in"=w648, "data"=FALSE) -> ("task out"=w646:refnum<k24>, "error out"=w645:errorcluster)  [unwired: 11 in, 1 out]
                  }
                  frame #1 {
                    n281 = Wait (ms)(milliseconds to wait=u32 4000) -> ()  [unwired: 1 out]
                  }
                  frame #2 {
                    # "turn on the display"
                    n282 = call-poly <vilib>:"ULx Write.vi"("task in"=w655, "data"=TRUE, "error in"=w653) -> ("error out"=w652:errorcluster)  [unwired: 10 in, 2 out]
                  }
                }
              }
              frame Disabled {
              }
            }
            n283 = property class="Str"(reference=w631) -> (reference out=w635:refnum<vi>, "Value"=w633:string)  [unwired: 1 in, 1 out]
            n284 = Concatenate Strings(w633, "\r", "RE-BOOTING...\n" ("string")) -> (w634:string)
            n285 = property class="Str"(reference=w635, "Value"=w634) -> ()  [unwired: 1 in, 2 out]
          }
          frame "udp mode" {
            n286 = Unbundle By Name(w666) -> ("Console"=w661:refnum<vi>, "COM"=w664:refnum<visa-resource-name>)
            n287 = property class="Str"(reference=w661) -> (reference out=w658:refnum<vi>, "Value"=w660:string)  [unwired: 1 in, 1 out]
            n288 = while {
              shift-right: [w693] -> _
              shift-left: w664 -> [w690]
              tunnel: [w671] -> w665
              tunnel: [w686] -> w667
              tunnel: w661 -> [w672]
              i -> [w681]
              stop <- w684 stop-if-true
              # "Serial Write and Read Loop"
              n289 = property class="Instr"(reference=w690) -> (reference out=w689:refnum<visa-resource-name>, error out=w688:errorcluster, "Serial Settings:Number of Bytes at Serial Port"=w687:u32)  [unwired: 1 in]
              n290 = property class="Str"(reference=w672) -> (reference out=w679:refnum<vi>, "Value"=w676:string)  [unwired: 1 in, 1 out]
              n291 = Equal To 0?(x=w681) -> (x = 0?=w680:bool)
              n292 = VISA Read(VISA resource name=w689, byte count=w687, error in (no error)=w688) -> (VISA resource name out=w693:refnum<visa-resource-name>, read buffer=w675:string, error out=w692:errorcluster)  [unwired: 1 out]
              n293 = Concatenate Strings(w676, w675) -> (w677:string)
              n294 = call "Elapsed Time2"("Time Target (s)"=60.0, "Reset"=w680) -> ("Time has Elapsed"=w683:bool)  [unwired: 10 in, 7 out]
              n295 = call "Stall Data Flow.vim"("value in"=w692, "milliseconds to wait"=u32 1) -> ("value out"=w671:errorcluster)  [unwired: 1 out]
              n296 = property class="Str"(reference=w679, "Value"=w677) -> (reference out=w674:refnum<vi>)  [unwired: 1 in, 1 out]
              n297 = Match Pattern(string=w675, regular expression="ProbeTimeoutHappened") -> (offset past match=w691:i32)  [unwired: 1 in, 3 out]
              n298 = Greater Or Equal To 0?(x=w691) -> (x >= 0?=w686:bool)
              n299 = property class="Str"(reference=w674, "Text.Scroll Position"=u32 4294967295) -> ()  [unwired: 1 in, 2 out]
              n300 = Or(x=w671, y=w686) -> (x .or. y?=w685:bool)
              n301 = Or(x=w685, y=w683) -> (x .or. y?=w684:bool)
            }
            n302 = Concatenate Strings(w660, "\nWaiting for ProbeStart to be present on the screen..." ("string")) -> (w662:string)
            n303 = property class="Str"(reference=w658, "Value"=w662) -> ()  [unwired: 1 in, 2 out]
            n304 = property on="Status" class="Str"("Value"="Entrando en modo programación" ("Status"), "Text.FontSize"=u32 32 ("Text.Font:Size")) -> ()  [unwired: 2 in, 2 out]
            n305 = case shown="False" w667 {
              tunnel: w669 -> [w699 w702]
              tunnel: w665 -> [w697 w703]
              tunnel: [w696 w700] -> w663
              frame False {
                n306 = Enqueue Element At Opposite End(queue=w699, element="error", error in (no error)=w697) -> (error out=w696:errorcluster)  [unwired: 1 in, 2 out]
                n307 = call "Custom User Message.vi"("Button text (\"OK\")"="OK" ("Button text (\"OK\")"), "MSG"="\nLa palabra \"ProbeStart\" nunca apareció en la pantalla.\nSi todo se encuentra bien conectado, contacte\na su supervisor para averiguar como proceder\n") -> ()  [unwired: 9 in, 1 out]
              }
              frame True {
                n308 = Enqueue Element(queue=w702, element="send udp", error in (no error)=w703) -> (error out=w700:errorcluster)  [unwired: 1 in, 2 out]
              }
            }
          }
          frame "send udp" {
            w711 = u16 7948  # remote port
            w712 = u16 7777  # local port
            n309 = Unbundle By Name(w709) -> ("Board IP"=w708:string)
            n310 = String To IP(1:w708) -> (0:w715:u32)
            n311 = UDP Open(11:w712) -> (port=w714:refnum<k16>, 0:w713:errorcluster)  [unwired: 4 in, 1 out]
            n312 = UDP Write(address=w715, port or service name=w711, connection ID=w714, data in="Program", 8:w713) -> (error out=w716:errorcluster, 3:w717:refnum<k16>)  [unwired: 1 in]
            n313 = UDP Close(connection ID=w717, 8:w716) -> (error out=w705:errorcluster)  [unwired: 1 out]
            n314 = case shown="Error .." w705 {
              selector: w705 -> [w719 w722]
              tunnel: w706 -> [w721 w727]
              tunnel: [w718 w725] -> w704
              frame No Error {
                n315 = Enqueue Element(queue=w721, element="login", error in (no error)=w719) -> (error out=w718:errorcluster)  [unwired: 1 in, 2 out]
              }
              frame Error {
                n316 = Enqueue Element At Opposite End(queue=w727, element="error", error in (no error)=w722) -> (error out=w725:errorcluster)  [unwired: 1 in, 2 out]
                n317 = call "Custom User Message.vi"("Button text (\"OK\")"="OK" ("Button text (\"OK\")"), "MSG"="\nHubo un problema al intentar poner la placa\nen modo de programación la configuración UDP es:\nlocal port: 7777\nremote port: 7948") -> ()  [unwired: 9 in, 1 out]
              }
            }
          }
          frame "login" {
            n318 = Unbundle By Name(w736) -> ("Console"=w731:refnum<vi>, "COM"=w734:refnum<visa-resource-name>)
            n319 = property class="Str"(reference=w731) -> (reference out=w728:refnum<vi>, "Value"=w730:string)  [unwired: 1 in, 1 out]
            n320 = while {
              shift-right: [w761] -> _
              shift-left: w734 -> [w758]
              tunnel: [w760] -> w735
              tunnel: [w754] -> w737
              tunnel: w731 -> [w740]
              i -> [w749]
              stop <- w752 stop-if-true
              # "Serial Write and Read Loop"
              n321 = property class="Instr"(reference=w758) -> (reference out=w757:refnum<visa-resource-name>, error out=w756:errorcluster, "Serial Settings:Number of Bytes at Serial Port"=w755:u32)  [unwired: 1 in]
              n322 = property class="Str"(reference=w740) -> (reference out=w747:refnum<vi>, "Value"=w744:string)  [unwired: 1 in, 1 out]
              n323 = VISA Read(VISA resource name=w757, byte count=w755, error in (no error)=w756) -> (VISA resource name out=w761:refnum<visa-resource-name>, read buffer=w743:string, error out=w760:errorcluster)  [unwired: 1 out]
              n324 = Equal To 0?(x=w749) -> (x = 0?=w748:bool)
              n325 = Concatenate Strings(w744, w743) -> (w745:string)
              n326 = call "Elapsed Time3"("Time Target (s)"=60.0, "Reset"=w748) -> ("Time has Elapsed"=w751:bool)  [unwired: 10 in, 7 out]
              n327 = property class="Str"(reference=w747, "Value"=w745) -> (reference out=w742:refnum<vi>)  [unwired: 1 in, 1 out]
              n328 = Match Pattern(string=w743, regular expression="Freescale Semiconductor") -> (offset past match=w759:i32)  [unwired: 1 in, 3 out]
              n329 = Greater Or Equal To 0?(x=w759) -> (x >= 0?=w754:bool)
              n330 = property class="Str"(reference=w742, "Text.Scroll Position"=u32 4294967295) -> ()  [unwired: 1 in, 2 out]
              n331 = Or(x=w760, y=w754) -> (x .or. y?=w753:bool)
              n332 = Or(x=w753, y=w751) -> (x .or. y?=w752:bool)
            }
            n333 = Concatenate Strings(w730, "\nWaiting for \"freescale\" to be present on the screen..." ("string")) -> (w732:string)
            n334 = property class="Str"(reference=w728, "Value"=w732) -> ()  [unwired: 1 in, 2 out]
            n335 = case shown="True" w737 {
              tunnel: w739 -> [w767 w780]
              tunnel: w735 -> [w765 w781]
              tunnel: [w764 w777] -> w733
              frame False {
                n336 = Enqueue Element At Opposite End(queue=w767, element="error", error in (no error)=w765) -> (error out=w764:errorcluster)  [unwired: 1 in, 2 out]
                n337 = call "Custom User Message.vi"("Button text (\"OK\")"="OK" ("Button text (\"OK\")"), "MSG"="\n\nSe ha perdido la conexión con el GUI\n") -> ()  [unwired: 9 in, 1 out]
              }
              frame True {
                n338 = Enqueue Element At Opposite End(queue=w780, element="flush", error in (no error)=w781) -> (queue out=w778:refnum<queue>, error out=w779:errorcluster)  [unwired: 1 in, 1 out]
                n339 = Enqueue Element(queue=w778, element="clear console", error in (no error)=w779) -> (queue out=w774:refnum<queue>, error out=w775:errorcluster)  [unwired: 1 in, 1 out]
                n340 = Enqueue Element(queue=w774, element="close visa", error in (no error)=w775) -> (queue out=w771:refnum<queue>, error out=w768:errorcluster)  [unwired: 1 in, 1 out]
                n341 = Enqueue Element(queue=w771, element="delay", error in (no error)=w768) -> (queue out=w769:refnum<queue>, error out=w770:errorcluster)  [unwired: 1 in, 1 out]
                n342 = Enqueue Element(queue=w769, element="prepare gui", error in (no error)=w770) -> (error out=w777:errorcluster)  [unwired: 1 in, 2 out]
              }
            }
          }
          frame "ping gui" {
            n343 = Unbundle By Name(w800) -> ("Console"=w799:refnum<vi>, "Board IP"=w786:string)
            n344 = property class="Str"(reference=w799) -> (reference out=w795:refnum<vi>, "Value"=w793:string)  [unwired: 1 in, 1 out]
            n345 = call <vilib>:"Space Constant.vi"() -> ("String"=w787:string)
            n346 = Concatenate Strings(w793, "\nPing-ing board...\n" ("string")) -> (w794:string)
            n347 = Concatenate Strings("ping -n 2" ("command line"), w787, w786) -> (w785:string)
            n348 = property class="Str"(reference=w795, "Value"=w794) -> (reference out=w791:refnum<vi>)  [unwired: 1 in, 1 out]
            n349 = call <vilib>:"System Exec.vi"("run minimized? (F)"=TRUE, "error in (no error)"=w810, "command line"=w785) -> ("error out"=w805:errorcluster, "standard error"=w807:string, "standard output"=w808:string)  [unwired: 5 in, 1 out]
            n350 = property class="Str"(reference=w791) -> (reference out=w789:refnum<vi>, "Value"=w790:string)  [unwired: 1 in, 1 out]
            n351 = Concatenate Strings(w808, w807) -> (w798:string)
            n352 = Concatenate Strings(w790, w798, "\r") -> (w797:string)
            n353 = disable-structure "Conditional Disable Structure" shown="Default" {
              disable-tunnel: ["perdidos = 0" "Received = 0"] -> w784
              frame condition #0 (active) {
              }
              frame condition #1 {
              }
            }
            n354 = property class="Str"(reference=w789, "Value"=w797) -> ()  [unwired: 1 in, 2 out]
            n355 = Match Pattern(string=w798, regular expression=w784) -> (offset past match=w809:i32)  [unwired: 1 in, 3 out]
            n356 = Greater Or Equal To 0?(x=w809) -> (x >= 0?=w806:bool)
            n357 = case shown="True" w806 {
              tunnel: w805 -> [w814 w830]
              tunnel: w804 -> [w815 w828]
              tunnel: [w813 w829] -> w803
              frame False {
                n358 = disable-structure shown="Enabled" {
                  disable-tunnel: w815 -> [w822 w824]
                  disable-tunnel: w814 -> [w821 w826]
                  disable-tunnel: [w818 w825] -> w813
                  frame Disabled {
                    n359 = Enqueue Element(queue=w822, element="reboot", error in (no error)=w821) -> (queue out=w817:refnum<queue>, error out=w819:errorcluster)  [unwired: 1 in, 1 out]
                    n360 = Enqueue Element(queue=w817, element="prepare gui", error in (no error)=w819) -> (error out=w818:errorcluster)  [unwired: 1 in, 2 out]
                  }
                  frame Enabled {
                    n361 = Enqueue Element(queue=w824, element="prepare gui", error in (no error)=w826) -> (error out=w825:errorcluster)  [unwired: 1 in, 2 out]
                  }
                }
              }
              frame True {
                n362 = call "Custom User Message.vi"("Button text (\"OK\")"="OK" ("Button text (\"OK\")"), "MSG"="Parece que hay un problema \ncon la configuración Ethernet\n asegúrese que:\nel IP: 10.134.246.249, y\nMask: 255.255.255.248\n") -> ()  [unwired: 9 in, 1 out]
                n363 = Enqueue Element At Opposite End(queue=w828, element="error", error in (no error)=w830) -> (error out=w829:errorcluster)  [unwired: 1 in, 2 out]
              }
            }
          }
          frame "prepare gui" {
            n364 = Unbundle By Name(w836) -> ("Console"=w846:refnum<vi>)
            n365 = property class="Str"(reference=w846) -> (reference out=w845:refnum<vi>, "Value"=w843:string)  [unwired: 1 in, 1 out]
            n366 = property on="Status" class="Str"("Value"="Programando GUI" ("Status"), "Text.FontSize"=u32 42 ("Text.Font:Size")) -> ()  [unwired: 2 in, 2 out]
            n367 = Unbundle By Name(w836) -> ("Android path"=w856:path)
            n368 = Concatenate Strings(w843, "\n>Preparing the GUI...\n" ("Value")) -> (w844:string)
            n369 = property class="Str"(reference=w845, "Value"=w844) -> (reference out=w847:refnum<vi>)  [unwired: 1 in, 1 out]
            n370 = call <vilib>:"System Exec.vi"("run minimized? (F)"=TRUE, "working directory"=w856, "command line"="python prepare_gui_board_labview.py") -> ("standard error"=w857:string, "standard output"=w855:string)  [unwired: 5 in, 2 out]
            n371 = call "Progress bar.vi"("TIme (s)"=250.0, "Title"="Preparing GUI") -> ()  [unwired: 9 in, 1 out]
            n372 = property class="Str"(reference=w847) -> (reference out=w860:refnum<vi>, "Value"=w861:string)  [unwired: 1 in, 1 out]
            n373 = Concatenate Strings(w861, w855, w857) -> (w859:string)
            n374 = property class="Str"(reference=w860, "Value"=w859) -> (reference out=w841:refnum<vi>, error out=w840:errorcluster)  [unwired: 1 in]
            n375 = Match Pattern(string=w855, regular expression="Watch display and make sure Tablo logo appears after a few minutes.") -> (offset past match=w853:i32)  [unwired: 1 in, 3 out]
            n376 = Greater Or Equal To 0?(x=w853) -> (x >= 0?=w851:bool)
            n377 = property class="Str"(reference=w841, error in=w840, "Text.Scroll Position"=u32 4294967295) -> ()  [unwired: 2 out]
            n378 = case shown="False" w851 {
              tunnel: w852 -> [w873 w893]
              tunnel: w850 -> [w871 w898]
              tunnel: [w872 w902] -> w848
              tunnel: w836 -> [w866 w892]
              tunnel: [w870 w891] -> w835
              frame False {
                n379 = Unbundle By Name(w866) -> ("Attempts left"=w863:i32)
                n380 = call <vilib>:"Close Progress Bar.vi"() -> ("error out"=w867:errorcluster)  [unwired: 10 in, 1 out]
                n381 = call <vilib>:"Clear Errors.vi"("error in (no error)"=w867) -> ()  [unwired: 5 in, 2 out]
                n382 = Less Or Equal To 0?(x=w863) -> (x <= 0?=w864:bool)
                n383 = Decrement(x=w863) -> (x-1=w865:i32)
                n384 = case shown="False" w864 {
                  tunnel: w873 -> [w883 w889]
                  tunnel: [w880 w887] -> w872
                  tunnel: w871 -> [w882 w886]
                  frame False {
                    n385 = Enqueue Element(queue=w883, element="kill adb", error in (no error)=w882) -> (queue out=w881:refnum<queue>, error out=w877:errorcluster)  [unwired: 1 in, 1 out]
                    n386 = Enqueue Element(queue=w881, element="delay", error in (no error)=w877) -> (queue out=w878:refnum<queue>, error out=w876:errorcluster)  [unwired: 1 in, 1 out]
                    n387 = Enqueue Element(queue=w878, element="prepare gui", error in (no error)=w876) -> (error out=w880:errorcluster)  [unwired: 1 in, 2 out]
                  }
                  frame True {
                    n388 = Enqueue Element At Opposite End(queue=w889, element="error", error in (no error)=w886) -> (error out=w887:errorcluster)  [unwired: 1 in, 2 out]
                    n389 = call "Custom User Message.vi"("Button text (\"OK\")"="Abortar" ("Button text (\"OK\")"), "MSG"="Parece ser que hubo un error al conectarse con la placa.\n\nAsegurase que la placa esta bien alimentada, el cable Ethernet bien conectado, reinicie, y vuelva a intentarlo. " ("message")) -> ()  [unwired: 9 in, 1 out]
                  }
                }
                n390 = Bundle By Name(cluster=w866, "Error"="Error al pasar el archivo \"prepare_gui_board.py\"", "Pass?"="False", "Attempts left"=w865) -> (w870:T2)
              }
              frame True {
                n391 = call <vilib>:"Close Progress Bar.vi"() -> ("error out"=w899:errorcluster)  [unwired: 10 in, 1 out]
                n392 = call <vilib>:"Clear Errors.vi"("error in (no error)"=w899) -> ("error out"=w897:errorcluster)  [unwired: 5 in, 1 out]
                n393 = Merge Errors(w897, w898) -> (w894:errorcluster)
                n394 = Enqueue Element(queue=w893, element="clear console", error in (no error)=w894) -> (queue out=w901:refnum<queue>, error out=w900:errorcluster)  [unwired: 1 in, 1 out]
                n395 = Bundle By Name(cluster=w892, "Attempts left"=7) -> (w891:T2)
                n396 = Enqueue Element(queue=w901, element="adb version", error in (no error)=w900) -> (error out=w902:errorcluster)  [unwired: 1 in, 2 out]
              }
            }
          }
          frame "kill adb" {
            n397 = Unbundle By Name(w917) -> ("Console"=w911:refnum<vi>, "Android path"=w916:path)
            n398 = property class="Str"(reference=w911) -> (reference out=w910:refnum<vi>, "Value"=w908:string)  [unwired: 1 in, 1 out]
            n399 = Concatenate Strings(w908, "\n>Making sure adb is not running in the background " ("string")) -> (w907:string)
            n400 = property class="Str"(reference=w910, "Value"=w907) -> (reference out=w909:refnum<vi>)  [unwired: 1 in, 1 out]
            n401 = property class="Str"(reference=w909) -> (reference out=w905:refnum<vi>, "Value"=w914:string)  [unwired: 1 in, 1 out]
            n402 = call <vilib>:"System Exec.vi"("run minimized? (F)"=TRUE, "working directory"=w916, "command line"="taskkill /F /IM adb.exe") -> ("standard error"=w912:string, "standard output"=w913:string)  [unwired: 5 in, 2 out]
            n403 = Concatenate Strings(w914, w913, w912) -> (w904:string)
            n404 = property class="Str"(reference=w905, "Value"=w904) -> ()  [unwired: 1 in, 2 out]
          }
          frame "adb version" {
            w939 = "1.0.36"  # adb target version
            n405 = Unbundle By Name(w922) -> ("Console"=w932:refnum<vi>, "Version path"=w924:path)
            n406 = property class="Str"(reference=w932) -> (reference out=w928:refnum<vi>, "Value"=w931:string)  [unwired: 1 in, 1 out]
            n407 = property on="Status" class="Str"("Value"="ADB: version" ("Status"), "Text.FontSize"=u32 65 ("Text.Font:Size")) -> ()  [unwired: 2 in, 2 out]
            n408 = Concatenate Strings(w931, ">" ("string"), w929, "\r") -> (w926:string)
            n409 = property class="Str"(reference=w928, "Value"=w926) -> (reference out=w927:refnum<vi>)  [unwired: 1 in, 1 out]
            n410 = call <vilib>:"System Exec.vi"("run minimized? (F)"=TRUE, "working directory"=w924, "command line"=w929) -> ("standard error"=w935:string, "standard output"=w940:string)  [unwired: 5 in, 2 out]
            n411 = property class="Str"(reference=w927) -> (reference out=w944:refnum<vi>, error out=w941:errorcluster, "Value"=w943:string)  [unwired: 1 in]
            n412 = Match Pattern(string=w940, regular expression=w939) -> (offset past match=w938:i32)  [unwired: 1 in, 3 out]
            n413 = Concatenate Strings(w943, w940, w935) -> (w942:string)
            n414 = Greater Or Equal To 0?(x=w938) -> (x >= 0?=w937:bool)
            n415 = property class="Str"(reference=w944, error in=w941, "Value"=w942) -> ()  [unwired: 2 out]
            n416 = case shown="True" w937 {
              tunnel: w936 -> [w954 w958]
              tunnel: w934 -> [w951 w959]
              tunnel: [w952 w972] -> w933
              tunnel: w922 -> [w947 w971]
              tunnel: [w948 w971] -> w921
              frame False {
                n417 = call "Custom User Message.vi"("Button text (\"OK\")"="Abortar" ("Button text (\"OK\")"), "MSG"="Parece ser que la versión 1.0.36 del Android Debug Bridge (ADB) \nno se encuentra instalada.\n\nPor favor instale la versión correcta y vuelva a intentarlo. " ("message")) -> ()  [unwired: 9 in, 1 out]
                n418 = Enqueue Element At Opposite End(queue=w954, element="error", error in (no error)=w951) -> (error out=w952:errorcluster)  [unwired: 1 in, 2 out]
                n419 = Bundle By Name(cluster=w947, "Error"="Version de ADB incorrecta", "Pass?"="False") -> (w948:T2)
              }
              frame True {
                n420 = disable-structure shown="Enabled" {
                  frame Disabled {
                    n421 = call "Custom User Message.vi"("Button text (\"OK\")"="OK" ("Button text (\"OK\")"), "MSG"="REBOOTEEE") -> ()  [unwired: 9 in, 1 out]
                  }
                  frame Enabled {
                  }
                }
                n422 = Enqueue Element(queue=w958, element="setting visa", error in (no error)=w959) -> (queue out=w955:refnum<queue>, error out=w956:errorcluster)  [unwired: 1 in, 1 out]
                n423 = Enqueue Element(queue=w955, element="reboot", error in (no error)=w956) -> (queue out=w962:refnum<queue>, error out=w961:errorcluster)  [unwired: 1 in, 1 out]
                n424 = Enqueue Element(queue=w962, element="IPv6", error in (no error)=w961) -> (queue out=w967:refnum<queue>, error out=w966:errorcluster)  [unwired: 1 in, 1 out]
                n425 = Enqueue Element(queue=w967, element="clear console", error in (no error)=w966) -> (queue out=w964:refnum<queue>, error out=w965:errorcluster)  [unwired: 1 in, 1 out]
                n426 = Enqueue Element(queue=w964, element="adb connect", error in (no error)=w965) -> (queue out=w969:refnum<queue>, error out=w968:errorcluster)  [unwired: 1 in, 1 out]
                n427 = Enqueue Element(queue=w969, element="os build", error in (no error)=w968) -> (error out=w972:errorcluster)  [unwired: 1 in, 2 out]
              }
            }
          }
          frame "IPv6" {
            n428 = Unbundle By Name(w987) -> ("Console"=w982:refnum<vi>, "COM"=w985:refnum<visa-resource-name>)
            n429 = property class="Str"(reference=w982) -> (reference out=w979:refnum<vi>, "Value"=w981:string)  [unwired: 1 in, 1 out]
            n430 = while {
              shift-right: [w1014] -> _
              shift-left: w985 -> [w1011]
              tunnel: [w992] -> w986
              tunnel: [w1007] -> w988
              tunnel: w982 -> [w993]
              i -> [w1002]
              stop <- w1005 stop-if-true
              # "Serial Write and Read Loop"
              n431 = property class="Instr"(reference=w1011) -> (reference out=w1010:refnum<visa-resource-name>, error out=w1009:errorcluster, "Serial Settings:Number of Bytes at Serial Port"=w1008:u32)  [unwired: 1 in]
              n432 = property class="Str"(reference=w993) -> (reference out=w1000:refnum<vi>, "Value"=w997:string)  [unwired: 1 in, 1 out]
              n433 = Equal To 0?(x=w1002) -> (x = 0?=w1001:bool)
              n434 = VISA Read(VISA resource name=w1010, byte count=w1008, error in (no error)=w1009) -> (VISA resource name out=w1014:refnum<visa-resource-name>, read buffer=w996:string, error out=w1013:errorcluster)  [unwired: 1 out]
              n435 = Concatenate Strings(w997, w996) -> (w998:string)
              n436 = call "Elapsed Time"("Time Target (s)"=120.0, "Reset"=w1001) -> ("Time has Elapsed"=w1004:bool)  [unwired: 10 in, 7 out]
              n437 = call "Stall Data Flow.vim"("value in"=w1013, "milliseconds to wait"=u32 1) -> ("value out"=w992:errorcluster)  [unwired: 1 out]
              n438 = property class="Str"(reference=w1000, "Value"=w998) -> (reference out=w995:refnum<vi>)  [unwired: 1 in, 1 out]
              n439 = Match Pattern(string=w996, regular expression="IPv6 routers") -> (offset past match=w1012:i32)  [unwired: 1 in, 3 out]
              n440 = Greater Or Equal To 0?(x=w1012) -> (x >= 0?=w1007:bool)
              n441 = property class="Str"(reference=w995, "Text.Scroll Position"=u32 4294967295) -> ()  [unwired: 1 in, 2 out]
              n442 = Or(x=w992, y=w1007) -> (x .or. y?=w1006:bool)
              n443 = Or(x=w1006, y=w1004) -> (x .or. y?=w1005:bool)
            }
            n444 = Concatenate Strings(w981, "\nWaiting for IPv6 to be present on the screen..." ("string")) -> (w983:string)
            n445 = property class="Str"(reference=w979, "Value"=w983) -> ()  [unwired: 1 in, 2 out]
            n446 = property on="Status" class="Str"("Value"="Esperando a que IPv6 \naparezca en la pantalla" ("Status"), "Text.FontSize"=u32 32 ("Text.Font:Size")) -> ()  [unwired: 2 in, 2 out]
            n447 = case shown="True" w988 {
              tunnel: w990 -> [w1020 w1022]
              tunnel: w986 -> [w1018 w1025]
              tunnel: [w1017 w1023] -> w984
              frame False {
                n448 = Enqueue Element At Opposite End(queue=w1020, element="error", error in (no error)=w1018) -> (error out=w1017:errorcluster)  [unwired: 1 in, 2 out]
                n449 = call "Custom User Message.vi"("Button text (\"OK\")"="OK" ("Button text (\"OK\")"), "MSG"="\nLa palabra \"IPv6\" nunca apareció en la pantalla.\nSi todo se encuentra bien conectado, contacte\na su supervisor para averiguar como proceder\n") -> ()  [unwired: 9 in, 1 out]
              }
              frame True {
                n450 = Enqueue Element At Opposite End(queue=w1022, element="close visa", error in (no error)=w1025) -> (queue out=w1021:refnum<queue>, error out=w1024:errorcluster)  [unwired: 1 in, 1 out]
                n451 = Enqueue Element At Opposite End(queue=w1021, element="flush", error in (no error)=w1024) -> (error out=w1023:errorcluster)  [unwired: 1 in, 2 out]
              }
            }
          }
          frame "close visa" {
            n452 = Unbundle By Name(w1035) -> ("COM"=w1028:refnum<visa-resource-name>)
            n453 = VISA Clear(VISA resource name=w1028) -> (VISA resource name out=w1029:refnum<visa-resource-name>, error out=w1030:errorcluster)  [unwired: 1 in]
            n454 = VISA Close(VISA resource name=w1029, error in (no error)=w1030) -> (error out=w1031:errorcluster)
            n455 = Bundle By Name(cluster=w1035, "COM"=refnum<visa-resource-name> refnum) -> (w1034:T2)
          }
          frame "adb connect" {
            n456 = Unbundle By Name(w1044) -> ("Console"=w1049:refnum<vi>, "Version path"=w1042:path, "Board IP"=w1039:string)
            n457 = property class="Str"(reference=w1049) -> (reference out=w1050:refnum<vi>, "Value"=w1048:string)  [unwired: 1 in, 1 out]
            n458 = Concatenate Strings(w1048, "\n>Connecting to GUI board...\n") -> (w1047:string)
            n459 = property class="Str"(reference=w1050, "Value"=w1047) -> (reference out=w1045:refnum<vi>)  [unwired: 1 in, 1 out]
            n460 = property on="Status" class="Str"("Value"="ADB: Conectándose al GUI" ("Status"), "Text.FontSize"=u32 36 ("Text.Font:Size")) -> ()  [unwired: 2 in, 2 out]
            n461 = call <vilib>:"Space Constant.vi"() -> ("String"=w1040:string)
            n462 = Concatenate Strings("adb connect" ("command line"), w1040, w1039) -> (w1038:string)
            n463 = call <vilib>:"System Exec.vi"("run minimized? (F)"=TRUE, "working directory"=w1042, "command line"=w1038) -> ("standard error"=w1053:string, "standard output"=w1060:string)  [unwired: 5 in, 2 out]
            n464 = property class="Str"(reference=w1045) -> (reference out=w1064:refnum<vi>, error out=w1061:errorcluster, "Value"=w1063:string)  [unwired: 1 in]
            n465 = Concatenate Strings(w1063, w1060, w1053) -> (w1062:string)
            n466 = Match Pattern(string=w1060, regular expression="connected") -> (offset past match=w1058:i32)  [unwired: 1 in, 3 out]
            n467 = Greater Or Equal To 0?(x=w1058) -> (x >= 0?=w1057:bool)
            n468 = property class="Str"(reference=w1064, error in=w1061, "Value"=w1062) -> ()  [unwired: 2 out]
            n469 = case shown="False" w1057 {
              tunnel: w1056 -> [w1072 _]
              tunnel: [w1071 w1084] -> w1052
              tunnel: w1051 -> [w1070 w1084]
              tunnel: w1044 -> [w1068 w1083]
              tunnel: [w1067 w1083] -> w1043
              frame False {
                n470 = Unbundle By Name(w1068) -> ("Attempts left"=w1066:i32)
                n471 = Less Or Equal To 0?(x=w1066) -> (x <= 0?=w1069:bool)
                n472 = Decrement(x=w1066) -> (x-1=w1065:i32)
                n473 = case shown="False" w1069 {
                  tunnel: w1072 -> [w1078 w1081]
                  tunnel: [w1077 w1080] -> w1071
                  tunnel: w1070 -> [w1076 w1079]
                  frame False {
                    n474 = call "Stall Data Flow.vim"("value in"=w1076, "milliseconds to wait"=u32 1000) -> ("value out"=w1074:errorcluster)  [unwired: 1 out]
                    n475 = Enqueue Element At Opposite End(queue=w1078, element="adb connect", error in (no error)=w1074) -> (error out=w1077:errorcluster)  [unwired: 1 in, 2 out]
                  }
                  frame True {
                    n476 = Enqueue Element At Opposite End(queue=w1081, element="unable to connect", error in (no error)=w1079) -> (error out=w1080:errorcluster)  [unwired: 1 in, 2 out]
                  }
                }
                n477 = Bundle By Name(cluster=w1068, "Attempts left"=w1065) -> (w1067:T2)
              }
              frame True {
              }
            }
          }
          frame "unable to connect" {
            n478 = call "Two BTN Custom User Message.vi"("Option 2 (\"Stop\")"="Abortar" ("F button name (\"Cancel\")"), "Option 1 (\"OK\")"="Reintentar" ("T button name (\"OK\")"), "Message"="Parece ser que hubo un error al conectarse con la placa.\n\nAsegurase que la placa esta bien alimentada, el cable Ethernet bien conectado y presione Reintentar. " ("message")) -> ("Ok?"=w1087:bool)  [unwired: 8 in]
            n479 = case shown="False" w1087 {
              tunnel: w1093 -> [w1100 w1104]
              tunnel: [w1098 w1103] -> w1092
              tunnel: w1086 -> [w1097 w1101]
              tunnel: [w1096 w1101] -> w1085
              frame False {
                n480 = Enqueue Element At Opposite End(queue=w1100, element="error") -> (error out=w1098:errorcluster)  [unwired: 2 in, 2 out]
                n481 = Bundle By Name(cluster=w1097, "Error"="Error al conectarse a la placa vía ethernet", "Pass?"="False") -> (w1096:T2)
              }
              frame True {
                n482 = Enqueue Element At Opposite End(queue=w1104, element="adb connect") -> (error out=w1103:errorcluster)  [unwired: 2 in, 2 out]
              }
            }
          }
          frame "os build" {
            n483 = Unbundle By Name(w1109) -> ("Console"=w1118:refnum<vi>, "Version path"=w1113:path)
            n484 = property class="Str"(reference=w1118) -> (reference out=w1121:refnum<vi>, error out=w1119:errorcluster, "Value"=w1120:string)  [unwired: 1 in]
            n485 = Concatenate Strings(w1120, ">adb shell cat /system/build.prop\n") -> (w1117:string)
            n486 = property on="Status" class="Str"("Value"="Asegurando que: \noutset.osbuild=4.0.0.4" ("Status"), "Text.FontSize"=u32 32 ("Text.Font:Size")) -> ()  [unwired: 2 in, 2 out]
            n487 = property class="Str"(reference=w1121, error in=w1119, "Value"=w1117) -> (reference out=w1116:refnum<vi>)  [unwired: 1 out]
            n488 = call <vilib>:"System Exec.vi"("run minimized? (F)"=TRUE, "working directory"=w1113, "command line"="adb shell cat /system/build.prop") -> ("standard error"=w1110:string, "standard output"=w1132:string)  [unwired: 5 in, 2 out]
            n489 = property class="Str"(reference=w1116) -> (reference out=w1136:refnum<vi>, error out=w1133:errorcluster, "Value"=w1135:string)  [unwired: 1 in]
            n490 = Concatenate Strings(w1135, w1132, w1110) -> (w1134:string)
            n491 = Match Pattern(string=w1132, regular expression="outset.osbuild=4.0.0.4") -> (offset past match=w1130:i32)  [unwired: 1 in, 3 out]
            n492 = Greater Or Equal To 0?(x=w1130) -> (x >= 0?=w1129:bool)
            n493 = property class="Str"(reference=w1136, error in=w1133, "Value"=w1134) -> (reference out=w1123:refnum<vi>)  [unwired: 1 out]
            n494 = Match Pattern(string=w1110, regular expression="kill-server") -> (offset past match=w1112:i32)  [unwired: 1 in, 3 out]
            n495 = property class="Str"(reference=w1123, "Text.Scroll Position"=u32 4294967295) -> ()  [unwired: 1 in, 2 out]
            n496 = Greater Or Equal To 0?(x=w1112) -> (x >= 0?=w1107:bool)
            n497 = case shown="True" w1129 {
              tunnel: w1128 -> [w1141 w1167]
              tunnel: [w1140 w1166] -> w1125
              tunnel: w1124 -> [w1139 w1165]
              tunnel: w1107 -> [w1138 _]
              tunnel: w1109 -> [w1137 w1164]
              tunnel: [w1137 w1164] -> w1108
              frame False {
                n498 = case shown="False" w1138 {
                  tunnel: w1141 -> [w1146 w1160]
                  tunnel: [w1145 w1163] -> w1140
                  tunnel: w1139 -> [w1144 w1161]
                  frame False {
                    n499 = Enqueue Element(queue=w1146, element="error", error in (no error)=w1144) -> (error out=w1145:errorcluster)  [unwired: 1 in, 2 out]
                    n500 = call "Custom User Message.vi"("Button text (\"OK\")"="Abortar" ("Button text (\"OK\")"), "MSG"="Parece ser que la versión del \nSistema Operativo de la tableta (GUI)\nno es la 4.0.0.4.\n\n Comuníquese con su superior\npara saber como proceder." ("message")) -> ()  [unwired: 9 in, 1 out]
                  }
                  frame True {
                    n501 = Enqueue Element(queue=w1160, element="adb kill-server", error in (no error)=w1161) -> (queue out=w1154:refnum<queue>, error out=w1157:errorcluster)  [unwired: 1 in, 1 out]
                    n502 = Enqueue Element(queue=w1154, element="delay", error in (no error)=w1157) -> (queue out=w1155:refnum<queue>, error out=w1156:errorcluster)  [unwired: 1 in, 1 out]
                    n503 = Enqueue Element(queue=w1155, element="adb connect", error in (no error)=w1156) -> (queue out=w1149:refnum<queue>, error out=w1152:errorcluster)  [unwired: 1 in, 1 out]
                    n504 = Enqueue Element(queue=w1149, element="delay", error in (no error)=w1152) -> (queue out=w1150:refnum<queue>, error out=w1151:errorcluster)  [unwired: 1 in, 1 out]
                    n505 = Enqueue Element(queue=w1150, element="os build", error in (no error)=w1151) -> (error out=w1163:errorcluster)  [unwired: 1 in, 2 out]
                  }
                }
              }
              frame True {
                n506 = Enqueue Element(queue=w1167, element="check screen", error in (no error)=w1165) -> (error out=w1166:errorcluster)  [unwired: 1 in, 2 out]
              }
            }
          }
          frame "check screen" {
            n507 = property on="Status" class="Str"("Value"="Verificación de pantalla" ("Status"), "Text.FontSize"=u32 36 ("Text.Font:Size")) -> ()  [unwired: 2 in, 2 out]
            n508 = call "Two BTN User Message XL.vi"("Option 2 (\"Stop\")"="¡Abortar!" ("F button name (\"Cancel\")"), "Option 1 (\"OK\")"="¡Todo bien!" ("T button name (\"OK\")"), "Message"="\n\n\nRealice la siguiente verificación funcional de la pantalla táctil, toque cada esquina \ny verifique que aparecen los siguientes números en cada una de ellas:\n\n-superior izquierda: 0 (+40 / -0), 0 (+40 / -0)\n-inferior izquierda: 0 (+40 / -0), 768 (+0 / -40)\n-inferior derecha: 1024 (+0 / -40), 768 (+0 / -40)\n-superior derecha: 1024 (+0 / -40), 0 (+40 / -0)\n\nEl numero aparece en la parte inferior central de la pantalla en cada caso. \nSi el número no coincide favor de comunicarse con el supervisor o el ingeniero.") -> ("Ok?"=w1173:bool)  [unwired: 8 in]
            n509 = case shown="False" w1173 {
              tunnel: w1180 -> [w1188 w1194]
              tunnel: [w1186 w1193] -> w1178
              tunnel: w1177 -> [w1185 w1192]
              tunnel: w1172 -> [w1183 w1191]
              tunnel: [w1184 w1191] -> w1171
              frame False {
                n510 = Enqueue Element(queue=w1188, element="error", error in (no error)=w1185) -> (error out=w1186:errorcluster)  [unwired: 1 in, 2 out]
                n511 = Bundle By Name(cluster=w1183, "Error"="Fallo la verificación de la pantalla táctil", "Pass?"="False") -> (w1184:T2)
              }
              frame True {
                n512 = call "Stall Data Flow.vim"("value in"=w1192, "milliseconds to wait"=u32 1000) -> ("value out"=w1190:errorcluster)  [unwired: 1 out]
                n513 = Enqueue Element(queue=w1194, element="adb uninstall", error in (no error)=w1190) -> (error out=w1193:errorcluster)  [unwired: 1 in, 2 out]
              }
            }
          }
          frame "adb uninstall" {
            n514 = Unbundle By Name(w1203) -> ("Console"=w1210:refnum<vi>, "Version path"=w1204:path)
            n515 = property class="Str"(reference=w1210) -> (reference out=w1211:refnum<vi>, "Value"=w1209:string)  [unwired: 1 in, 1 out]
            n516 = Concatenate Strings(w1209, "\n>adb uninstall sequoia.gui.demo\n") -> (w1207:string)
            n517 = property on="Status" class="Str"("Value"="ADB: uninstall sequoia.gui.demo" ("Status"), "Text.FontSize"=u32 32 ("Text.Font:Size")) -> ()  [unwired: 2 in, 2 out]
            n518 = property class="Str"(reference=w1211, "Value"=w1207) -> (reference out=w1208:refnum<vi>)  [unwired: 1 in, 1 out]
            n519 = call <vilib>:"System Exec.vi"("run minimized? (F)"=TRUE, "working directory"=w1204, "command line"="adb uninstall sequoia.gui.demo") -> ("standard error"=w1201:string, "standard output"=w1222:string)  [unwired: 5 in, 2 out]
            n520 = property class="Str"(reference=w1208) -> (reference out=w1226:refnum<vi>, error out=w1223:errorcluster, "Value"=w1225:string)  [unwired: 1 in]
            n521 = Concatenate Strings(w1225, w1222, w1201) -> (w1224:string)
            n522 = Match Pattern(string=w1222, regular expression="Success") -> (offset past match=w1221:i32)  [unwired: 1 in, 3 out]
            n523 = Match Pattern(string=w1201, regular expression="kill-server") -> (offset past match=w1214:i32)  [unwired: 1 in, 3 out]
            n524 = Greater Or Equal To 0?(x=w1221) -> (x >= 0?=w1220:bool)
            n525 = Greater Or Equal To 0?(x=w1214) -> (x >= 0?=w1200:bool)
            n526 = property class="Str"(reference=w1226, error in=w1223, "Value"=w1224) -> (reference out=w1197:refnum<vi>)  [unwired: 1 out]
            n527 = property class="Str"(reference=w1197, "Text.Scroll Position"=u32 4294967295) -> ()  [unwired: 1 in, 2 out]
            n528 = case shown="True" w1220 {
              tunnel: w1219 -> [w1232 w1257]
              tunnel: w1200 -> [w1231 _]
              tunnel: [w1230 w1253] -> w1213
              tunnel: w1212 -> [w1229 w1252]
              tunnel: w1203 -> [w1228 w1251]
              tunnel: [w1227 w1251] -> w1202
              frame False {
                n529 = case shown="False" w1231 {
                  tunnel: w1232 -> [w1241 w1250]
                  tunnel: [w1240 w1245] -> w1230
                  tunnel: w1229 -> [w1239 w1248]
                  tunnel: w1228 -> [w1236 w1247]
                  tunnel: [w1235 w1247] -> w1227
                  frame False {
                    n530 = call "Custom User Message.vi"("Button text (\"OK\")"="Abortar" ("Button text (\"OK\")"), "MSG"="------------------------------\nError: \nfailed to uninstall \nsequioa.gui.demo\n------------------------------") -> ()  [unwired: 9 in, 1 out]
                    n531 = Enqueue Element(queue=w1241, element="error", error in (no error)=w1239) -> (error out=w1240:errorcluster)  [unwired: 1 in, 2 out]
                    n532 = Bundle By Name(cluster=w1236, "Error"="Error al instalar \"sequioa.gui.demo\"", "Pass?"="False") -> (w1235:T2)
                  }
                  frame True {
                    n533 = Enqueue Element(queue=w1250, element="adb kill-server", error in (no error)=w1248) -> (queue out=w1244:refnum<queue>, error out=w1246:errorcluster)  [unwired: 1 in, 1 out]
                    n534 = Enqueue Element(queue=w1244, element="adb uninstall", error in (no error)=w1246) -> (error out=w1245:errorcluster)  [unwired: 1 in, 2 out]
                  }
                }
              }
              frame True {
                n535 = call "Stall Data Flow.vim"("value in"=w1257, "milliseconds to wait"=u32 1000) -> ("value out"=w1255:refnum<queue>)  [unwired: 1 out]
                n536 = Enqueue Element(queue=w1255, element="adb install", error in (no error)=w1252) -> (error out=w1253:errorcluster)  [unwired: 1 in, 2 out]
              }
            }
          }
          frame "adb kill-server" {
            n537 = Unbundle By Name(w1258) -> ("Console"=w1267:refnum<vi>, "Version path"=w1260:path)
            n538 = property class="Str"(reference=w1267) -> (reference out=w1266:refnum<vi>, "Value"=w1265:string)  [unwired: 1 in, 1 out]
            n539 = Concatenate Strings(w1265, "\n>adb kill-server\n") -> (w1264:string)
            n540 = property class="Str"(reference=w1266, "Value"=w1264) -> (reference out=w1262:refnum<vi>)  [unwired: 1 in, 1 out]
            n541 = call <vilib>:"System Exec.vi"("run minimized? (F)"=TRUE, "working directory"=w1260, "command line"=w1268) -> ("error out"=w1259:errorcluster, "standard error"=w1269:string, "standard output"=w1270:string)  [unwired: 5 in, 1 out]
            n542 = property class="Str"(reference=w1262) -> (reference out=w1274:refnum<vi>, error out=w1271:errorcluster, "Value"=w1273:string)  [unwired: 1 in]
            n543 = Concatenate Strings(w1273, w1270, w1269) -> (w1272:string)
            n544 = property class="Str"(reference=w1274, error in=w1271, "Value"=w1272) -> ()  [unwired: 2 out]
          }
          frame "adb install" {
            n545 = Unbundle By Name(w1278) -> ("Console"=w1287:refnum<vi>, "Version path"=w1279:path)
            n546 = property class="Str"(reference=w1287) -> (reference out=w1288:refnum<vi>, "Value"=w1284:string)  [unwired: 1 in, 1 out]
            n547 = Concatenate Strings(w1284, "\n>adb install -r SequoiaGUI.apk\n") -> (w1285:string)
            n548 = property on="Status" class="Str"("Value"="ADB: install SequoiaGUI.apk" ("Status"), "Text.FontSize"=u32 32 ("Text.Font:Size")) -> ()  [unwired: 2 in, 2 out]
            n549 = property class="Str"(reference=w1288, "Value"=w1285) -> (reference out=w1286:refnum<vi>)  [unwired: 1 in, 1 out]
            n550 = call <vilib>:"System Exec.vi"("run minimized? (F)"=TRUE, "working directory"=w1279, "command line"="adb install -r SequoiaGUI.apk") -> ("standard error"=w1290:string, "standard output"=w1297:string)  [unwired: 5 in, 2 out]
            n551 = property class="Str"(reference=w1286) -> (reference out=w1301:refnum<vi>, error out=w1298:errorcluster, "Value"=w1300:string)  [unwired: 1 in]
            n552 = Concatenate Strings(w1300, w1297, w1290) -> (w1299:string)
            n553 = Match Pattern(string=w1297, regular expression="Success") -> (offset past match=w1295:i32)  [unwired: 1 in, 3 out]
            n554 = Greater Or Equal To 0?(x=w1295) -> (x >= 0?=w1294:bool)
            n555 = property class="Str"(reference=w1301, error in=w1298, "Value"=w1299) -> (reference out=w1280:refnum<vi>)  [unwired: 1 out]
            n556 = property class="Str"(reference=w1280, "Text.Scroll Position"=u32 4294967295) -> ()  [unwired: 1 in, 2 out]
            n557 = case shown="True" w1294 {
              tunnel: w1293 -> [w1309 w1318]
              tunnel: [w1308 w1315] -> w1289
              tunnel: w1278 -> [w1305 w1312]
              tunnel: [w1304 w1311] -> w1277
              frame False {
                n558 = call "Custom User Message.vi"("Button text (\"OK\")"="Abortar" ("Button text (\"OK\")"), "MSG"="------------------------------\nError: \nunhandle excepcion in \nadb install\n------------------------------") -> ()  [unwired: 9 in, 1 out]
                n559 = Enqueue Element(queue=w1309, element="error") -> (error out=w1308:errorcluster)  [unwired: 2 in, 2 out]
                n560 = Bundle By Name(cluster=w1305, "Error"="Error al instalar \"SequoiaGUI.apk\"", "Pass?"="False") -> (w1304:T2)
              }
              frame True {
                (unwired) "adb reboot" ("element")
                n561 = call "Stall Data Flow.vim"("value in"=w1318, "milliseconds to wait"=u32 500) -> ("value out"=w1317:refnum<queue>)  [unwired: 1 out]
                n562 = Bundle By Name(cluster=w1312, "Attempts left"=3) -> (w1311:T2)
                n563 = Enqueue Element(queue=w1317, element="update media") -> (error out=w1315:errorcluster)  [unwired: 2 in, 2 out]
              }
            }
          }
          frame "adb reboot" {
            n564 = Unbundle By Name(w1321) -> ("Console"=w1329:refnum<vi>, "Version path"=w1322:path)
            n565 = property class="Str"(reference=w1329) -> (reference out=w1331:refnum<vi>, error out=w1332:errorcluster, "Value"=w1328:string)  [unwired: 1 in]
            n566 = property on="Status" class="Str"("Value"="ADB: reboot" ("Status"), "Text.FontSize"=u32 60 ("Text.Font:Size")) -> ()  [unwired: 2 in, 2 out]
            n567 = Concatenate Strings(w1328, "\n>adb reboot\n" ("string")) -> (w1327:string)
            n568 = property class="Str"(reference=w1331, error in=w1332, "Value"=w1327) -> (reference out=w1330:refnum<vi>)  [unwired: 1 out]
            n569 = call <vilib>:"System Exec.vi"("run minimized? (F)"=TRUE, "working directory"=w1322, "command line"=w1345) -> ("error out"=w1340:errorcluster, "standard error"=w1343:string, "standard output"=w1344:string)  [unwired: 5 in, 1 out]
            n570 = property class="Str"(reference=w1330) -> (reference out=w1351:refnum<vi>, error out=w1348:errorcluster, "Value"=w1350:string)  [unwired: 1 in]
            n571 = call "Stall Data Flow.vim"("value in"=w1340, "milliseconds to wait"=u32 1000) -> ("value out"=w1339:errorcluster)  [unwired: 1 out]
            n572 = Concatenate Strings(w1350, w1344, w1343) -> (w1349:string)
            n573 = property class="Str"(reference=w1351, error in=w1348, "Value"=w1349) -> ()  [unwired: 2 out]
            n574 = Enqueue Element(queue=w1347, element="clear console") -> (queue out=w1325:refnum<queue>)  [unwired: 2 in, 2 out]
            n575 = Enqueue Element(queue=w1325, element="reboot", error in (no error)=w1339) -> (queue out=w1342:refnum<queue>, error out=w1337:errorcluster)  [unwired: 1 in, 1 out]
            n576 = Enqueue Element(queue=w1342, element="delay", error in (no error)=w1337) -> (queue out=w1336:refnum<queue>, error out=w1334:errorcluster)  [unwired: 1 in, 1 out]
            n577 = Enqueue Element(queue=w1336, element="update media", error in (no error)=w1334) -> (error out=w1333:errorcluster)  [unwired: 1 in, 2 out]
          }
          frame "delay" {
            w1354 = "\r"
            n578 = Unbundle By Name(w1359) -> ("Console"=w1358:refnum<vi>)
            n579 = property class="Str"(reference=w1358) -> (reference out=w1357:refnum<vi>, "Value"=w1355:string)  [unwired: 1 in, 1 out]
            n580 = Concatenate Strings(w1355, w1354, w1354, "." ("string")) -> (w1356:string)
            n581 = property class="Str"(reference=w1357, "Value"=w1356) -> (reference out=w1352:refnum<vi>)  [unwired: 1 in, 1 out]
            n582 = for {
              N: 4 -> [_]
              shift-right: [w1370] -> w1360
              shift-left: w1361 -> [w1371]
              tunnel: w1352 -> [w1366]
              n583 = property class="Str"(reference=w1366) -> (reference out=w1368:refnum<vi>, "Value"=w1367:string)  [unwired: 1 in, 1 out]
              n584 = call "Stall Data Flow.vim"("value in"=w1371, "milliseconds to wait"=u32 500) -> ("value out"=w1370:errorcluster)  [unwired: 1 out]
              n585 = Concatenate Strings(w1367, "...") -> (w1364:string)
              n586 = property class="Str"(reference=w1368, "Value"=w1364) -> ()  [unwired: 1 in, 2 out]
            }
          }
          frame "update media" {
            n587 = Unbundle By Name(w1376) -> ("Console"=w1390:refnum<vi>, "Python 2.7"=w1377:path)
            n588 = Open Python Session(python version="2.7.11" ("Python version"), python path=w1377, 3:w1382) -> (session out=w1375:refnum<k35>, error out=w1381:errorcluster)
            n589 = property on="Status" class="Str"("Value"="Actualizando archivos multimedia" ("Status"), "Text.FontSize"=u32 32 ("Text.Font:Size")) -> ()  [unwired: 2 in, 2 out]
            n590 = property class="Str"(reference=w1390) -> (reference out=w1389:refnum<vi>, error out=w1386:errorcluster, "Value"=w1388:string)  [unwired: 1 in]
            n591 = Concatenate Strings(w1388, "\n>Opening Update_Media_Labview.py session...") -> (w1387:string)
            n592 = property class="Str"(reference=w1389, error in=w1386, "Value"=w1387) -> (reference out=w1378:refnum<vi>)  [unwired: 1 out]
            n593 = case shown="No Error" w1381 {
              selector: w1381 -> [w1402 w1412]
              tunnel: w1380 -> [w1403 w1413]
              tunnel: [w1400 w1411] -> w1379
              tunnel: w1378 -> [w1395 _]
              tunnel: w1376 -> [w1393 w1407]
              tunnel: w1375 -> [w1392 _]
              tunnel: [w1391 w1406] -> w1374
              frame No Error {
                n594 = property class="Str"(reference=w1395) -> (reference out=w1399:refnum<vi>, error out=w1396:errorcluster, "Value"=w1398:string)  [unwired: 1 in]
                n595 = Bundle By Name(cluster=w1393, "Python session"=w1392) -> (w1391:T2)
                n596 = Concatenate Strings(w1398, "\nOK" ("string")) -> (w1397:string)
                n597 = Enqueue Element(queue=w1403, element="ensure temp dir", error in (no error)=w1402) -> (error out=w1400:errorcluster)  [unwired: 1 in, 2 out]
                n598 = property class="Str"(reference=w1399, error in=w1396, "Value"=w1397) -> ()  [unwired: 2 out]
              }
              frame Error {
                n599 = call "Custom User Message.vi"("Button text (\"OK\")"="Abortar" ("Button text (\"OK\")"), "MSG"="Parece ser que la versión 2.7.11 de Python \nno se encuentra instalada.\n\nPor favor instale la versión correcta y vuelva a intentar. " ("message")) -> ()  [unwired: 9 in, 1 out]
                n600 = Enqueue Element(queue=w1413, element="error", error in (no error)=w1412) -> (error out=w1411:errorcluster)  [unwired: 1 in, 2 out]
                n601 = Bundle By Name(cluster=w1407, "Error"="Version incorrecta de python", "Pass?"="False") -> (w1406:T2)
              }
            }
          }
          frame "ensure temp dir" {
            n602 = Unbundle By Name(w1417) -> ("Console"=w1414:refnum<vi>, "Python session"=w1423:refnum<k35>, "Script path"=w1422:path)
            n603 = node(w1423, w1422, "ensure_temp_dir" ("function name"), w1421) -> (w1420:errorcluster)  [unwired: 2 in, 3 out]
            n604 = property class="Str"(reference=w1414) -> (reference out=w1429:refnum<vi>, error out=w1426:errorcluster, "Value"=w1428:string)  [unwired: 1 in]
            n605 = Concatenate Strings(w1428, "\n>Looking for temp directory...\n " ("function name")) -> (w1427:string)
            n606 = property class="Str"(reference=w1429, error in=w1426, "Value"=w1427) -> (reference out=w1415:refnum<vi>)  [unwired: 1 out]
            n607 = case shown="No Error" w1420 {
              selector: w1420 -> [w1444 w1449]
              tunnel: w1418 -> [w1445 w1447]
              tunnel: [w1442 w1448] -> w1419
              tunnel: w1415 -> [w1431 _]
              frame No Error {
                n608 = property class="Str"(reference=w1431) -> (reference out=w1435:refnum<vi>, error out=w1432:errorcluster, "Value"=w1434:string)  [unwired: 1 in]
                n609 = Enqueue Element(queue=w1445, element="adb connect", error in (no error)=w1444) -> (queue out=w1441:refnum<queue>, error out=w1438:errorcluster)  [unwired: 1 in, 1 out]
                n610 = Concatenate Strings(w1434, "Finded!" ("string")) -> (w1433:string)
                n611 = Enqueue Element(queue=w1441, element="clear console", error in (no error)=w1438) -> (queue out=w1439:refnum<queue>, error out=w1437:errorcluster)  [unwired: 1 in, 1 out]
                n612 = property class="Str"(reference=w1435, error in=w1432, "Value"=w1433) -> ()  [unwired: 2 out]
                n613 = Enqueue Element(queue=w1439, element="media required", error in (no error)=w1437) -> (error out=w1442:errorcluster)  [unwired: 1 in, 2 out]
              }
              frame Error {
                n614 = Enqueue Element(queue=w1447, element="error", error in (no error)=w1449) -> (error out=w1448:errorcluster)  [unwired: 1 in, 2 out]
              }
            }
          }
          frame "media required" {
            n615 = Unbundle By Name(w1452) -> ("Console"=w1456:refnum<vi>, "Python session"=w1467:refnum<k35>, "Script path"=w1466:path)
            n616 = property class="Str"(reference=w1456) -> (reference out=w1473:refnum<vi>, error out=w1470:errorcluster, "Value"=w1472:string)  [unwired: 1 in]
            n617 = Concatenate Strings(w1472, ">Looking for media required...\n" ("function name")) -> (w1471:string)
            n618 = property class="Str"(reference=w1473, error in=w1470, "Value"=w1471) -> (reference out=w1459:refnum<vi>, error out=w1455:errorcluster)
            n619 = call "Stall Data Flow.vim"("value in"=w1455, "milliseconds to wait"=u32 500) -> ("value out"=w1454:errorcluster)  [unwired: 1 out]
            n620 = node(w1467, w1466, "get_media_required" ("function name"), w1454, cluster{i32, string} {0, ""}) -> (w1451:refnum<k35>, w1465:errorcluster, w1461:cluster{i32, string})  [unwired: 2 out]
            n621 = Unbundle(w1461) -> (w1457:i32, w1458:string)
            n622 = case shown="No Error" w1465 {
              selector: w1465 -> [w1491 w1502]
              tunnel: w1463 -> [w1492 w1500]
              tunnel: [w1490 w1501] -> w1464
              tunnel: w1459 -> [w1485 _]
              tunnel: w1458 -> [w1477 _]
              tunnel: w1457 -> [w1478 _]
              tunnel: w1452 -> [w1479 w1496]
              tunnel: w1451 -> [w1476 _]
              tunnel: [w1475 w1495] -> w1450
              frame No Error {
                n623 = property class="Str"(reference=w1485) -> (reference out=w1489:refnum<vi>, error out=w1486:errorcluster, "Value"=w1488:string)  [unwired: 1 in]
                n624 = Number To Decimal String(number=w1478) -> (decimal integer string=w1481:string)  [unwired: 1 in]
                n625 = Bundle By Name(cluster=w1479, "Media version"=w1478, "Media Url"=w1477, "Python session"=w1476) -> (w1475:T2)
                n626 = Concatenate Strings(w1488, "Url: " ("string"), w1477, "\r", "Version: #" ("string"), w1481, "\r") -> (w1487:string)
                n627 = property class="Str"(reference=w1489, error in=w1486, "Value"=w1487) -> ()  [unwired: 2 out]
                n628 = Enqueue Element(queue=w1492, element="media exist?", error in (no error)=w1491) -> (error out=w1490:errorcluster)  [unwired: 1 in, 2 out]
              }
              frame Error {
                n629 = call "Custom User Message.vi"("Button text (\"OK\")"="Abortar" ("Button text (\"OK\")"), "MSG"="------------------------------------\nFatal error opening labview script\n------------------------------------" ("message")) -> ()  [unwired: 9 in, 1 out]
                n630 = Bundle By Name(cluster=w1496, "Error"="Error abriendo labview script", "Pass?"="False") -> (w1495:T2)
                n631 = Enqueue Element(queue=w1500, element="error", error in (no error)=w1502) -> (error out=w1501:errorcluster)  [unwired: 1 in, 2 out]
              }
            }
          }
          frame "media exist?" {
            n632 = Unbundle By Name(w1503) -> ("Media version"=w1511:i32)
            n633 = Number To Decimal String(number=w1511) -> (decimal integer string=w1513:string)  [unwired: 1 in]
            n634 = Concatenate Strings(w1513, ".zip" ("string")) -> (w1514:string)
            n635 = String To Path(string=w1514) -> (path=w1510:path)
            n636 = Build Path(base path=path "C:/GUIMedia", name or relative path=w1510) -> (appended path=w1509:path)
            n637 = call <vilib>:"Check if File or Folder Exists.vi"("path"=w1509) -> ("file or folder exists?"=w1508:bool)  [unwired: 8 in, 2 out]
            n638 = case shown="True" w1508 {
              tunnel: w1507 -> [w1517 w1521]
              tunnel: w1506 -> [w1519 w1523]
              tunnel: [w1516 w1520] -> w1504
              frame True {
                n639 = Enqueue Element(queue=w1517, element="rm media", error in (no error)=w1519) -> (error out=w1516:errorcluster)  [unwired: 1 in, 2 out]
              }
              frame False {
                n640 = Enqueue Element(queue=w1521, element="download", error in (no error)=w1523) -> (error out=w1520:errorcluster)  [unwired: 1 in, 2 out]
              }
            }
          }
          frame "download" {
            n641 = Unbundle By Name(w1532) -> ("Version path"=w1531:path)
            n642 = flat-sequence {
              tunnel: w1531 -> [w1536]
              tunnel: w1527 -> [w1533]
              tunnel: [w1533] -> w1526
              tunnel: w1526 -> [w1539]
              tunnel: [w1539] -> w1525
              frame #0 {
                n643 = call <vilib>:"System Exec.vi"("wait until completion? (T)"=FALSE, "working directory"=w1536, "command line"="python Update_Media.py") -> ()  [unwired: 5 in, 4 out]
              }
              frame #1 {
                n644 = call "Custom User Message.vi"("Button text (\"OK\")"="Continuar" ("button name (\"OK\")"), "MSG"="\n\nEspere a termine el script y presione continuar..." ("message")) -> ()  [unwired: 9 in, 1 out]
              }
            }
            n645 = Enqueue Element(queue=w1525, element="end", error in (no error)=w1529) -> (error out=w1528:errorcluster)  [unwired: 1 in, 2 out]
          }
          frame "rm media" {
            n646 = Unbundle By Name(w1541) -> ("Console"=w1549:refnum<vi>, "Version path"=w1542:path)
            n647 = property class="Str"(reference=w1549) -> (reference out=w1550:refnum<vi>, "Value"=w1548:string)  [unwired: 1 in, 1 out]
            n648 = Concatenate Strings(w1548, "\n>rm -r -f /sdcard/media\n") -> (w1547:string)
            n649 = property class="Str"(reference=w1550, "Value"=w1547) -> (reference out=w1545:refnum<vi>)  [unwired: 1 in, 1 out]
            n650 = call <vilib>:"System Exec.vi"("run minimized? (F)"=TRUE, "working directory"=w1542, "command line"="adb shell rm -r -f /sdcard/media") -> ("error out"=w1544:errorcluster, "standard error"=w1552:string, "standard output"=w1557:string)  [unwired: 5 in, 1 out]
            n651 = property class="Str"(reference=w1545) -> (reference out=w1561:refnum<vi>, error out=w1558:errorcluster, "Value"=w1560:string)  [unwired: 1 in]
            n652 = Concatenate Strings(w1560, w1557, w1552) -> (w1559:string)
            n653 = property class="Str"(reference=w1561, error in=w1558, "Value"=w1559) -> (reference out=w1543:refnum<vi>)  [unwired: 1 out]
            n654 = case shown="No Error" w1544 {
              selector: w1544 -> [w1569 w1577]
              tunnel: w1556 -> [w1572 _]
              tunnel: [w1571 w1577] -> w1551
              tunnel: w1543 -> [w1564 _]
              tunnel: w1541 -> [w1562 w1576]
              tunnel: [w1562 w1575] -> w1540
              frame No Error {
                n655 = property class="Str"(reference=w1564) -> (reference out=w1563:refnum<vi>, error out=w1568:errorcluster, "Value"=w1567:string)  [unwired: 1 in]
                n656 = Concatenate Strings(w1567, "Done!" ("string")) -> (w1566:string)
                n657 = property class="Str"(reference=w1563, error in=w1568, "Value"=w1566) -> ()  [unwired: 2 out]
                n658 = Enqueue Element At Opposite End(queue=w1572, element="mkdir media", error in (no error)=w1569) -> (error out=w1571:errorcluster)  [unwired: 1 in, 2 out]
              }
              frame Error {
                n659 = Bundle By Name(cluster=w1576, "Error"="Error al ejecutar el cmd shell", "Pass?"="False") -> (w1575:T2)
              }
            }
          }
          frame "mkdir media" {
            n660 = Unbundle By Name(w1579) -> ("Console"=w1587:refnum<vi>, "Version path"=w1580:path)
            n661 = property class="Str"(reference=w1587) -> (reference out=w1588:refnum<vi>, "Value"=w1586:string)  [unwired: 1 in, 1 out]
            n662 = Concatenate Strings(w1586, "\n>mkdir /sdcard/media\n") -> (w1585:string)
            n663 = property class="Str"(reference=w1588, "Value"=w1585) -> (reference out=w1583:refnum<vi>)  [unwired: 1 in, 1 out]
            n664 = call <vilib>:"System Exec.vi"("run minimized? (F)"=TRUE, "working directory"=w1580, "command line"="adb shell mkdir /sdcard/media") -> ("error out"=w1582:errorcluster, "standard error"=w1590:string, "standard output"=w1595:string)  [unwired: 5 in, 1 out]
            n665 = property class="Str"(reference=w1583) -> (reference out=w1599:refnum<vi>, error out=w1596:errorcluster, "Value"=w1598:string)  [unwired: 1 in]
            n666 = Concatenate Strings(w1598, w1595, w1590) -> (w1597:string)
            n667 = property class="Str"(reference=w1599, error in=w1596, "Value"=w1597) -> (reference out=w1581:refnum<vi>)  [unwired: 1 out]
            n668 = case shown="No Error" w1582 {
              selector: w1582 -> [w1607 w1615]
              tunnel: w1594 -> [w1610 _]
              tunnel: [w1609 w1615] -> w1589
              tunnel: w1581 -> [w1602 _]
              tunnel: w1579 -> [w1600 w1612]
              tunnel: [w1600 w1611] -> w1578
              frame No Error {
                n669 = property class="Str"(reference=w1602) -> (reference out=w1601:refnum<vi>, error out=w1606:errorcluster, "Value"=w1605:string)  [unwired: 1 in]
                n670 = Concatenate Strings(w1605, "Done!" ("string")) -> (w1604:string)
                n671 = Enqueue Element At Opposite End(queue=w1610, element="mkdir temp", error in (no error)=w1607) -> (error out=w1609:errorcluster)  [unwired: 1 in, 2 out]
                n672 = property class="Str"(reference=w1601, error in=w1606, "Value"=w1604) -> ()  [unwired: 2 out]
              }
              frame Error {
                n673 = Bundle By Name(cluster=w1612, "Error"="Error al ejecutar el cmd shell", "Pass?"="False") -> (w1611:T2)
              }
            }
          }
          frame "mkdir temp" {
            n674 = Unbundle By Name(w1617) -> ("Console"=w1625:refnum<vi>, "Version path"=w1618:path)
            n675 = property class="Str"(reference=w1625) -> (reference out=w1626:refnum<vi>, "Value"=w1624:string)  [unwired: 1 in, 1 out]
            n676 = Concatenate Strings(w1624, "\n>adb shell mkdir /sdcard/media/temp\n") -> (w1623:string)
            n677 = property class="Str"(reference=w1626, "Value"=w1623) -> (reference out=w1621:refnum<vi>)  [unwired: 1 in, 1 out]
            n678 = call <vilib>:"System Exec.vi"("run minimized? (F)"=TRUE, "working directory"=w1618, "command line"="adb shell mkdir /sdcard/media/temp") -> ("error out"=w1620:errorcluster, "standard error"=w1628:string, "standard output"=w1633:string)  [unwired: 5 in, 1 out]
            n679 = property class="Str"(reference=w1621) -> (reference out=w1637:refnum<vi>, error out=w1634:errorcluster, "Value"=w1636:string)  [unwired: 1 in]
            n680 = Concatenate Strings(w1636, w1633, w1628) -> (w1635:string)
            n681 = property class="Str"(reference=w1637, error in=w1634, "Value"=w1635) -> (reference out=w1619:refnum<vi>)  [unwired: 1 out]
            n682 = case shown="No Error" w1620 {
              selector: w1620 -> [w1645 w1653]
              tunnel: w1632 -> [w1648 _]
              tunnel: [w1647 w1653] -> w1627
              tunnel: w1619 -> [w1640 _]
              tunnel: w1617 -> [w1638 w1650]
              tunnel: [w1638 w1649] -> w1616
              frame No Error {
                n683 = property class="Str"(reference=w1640) -> (reference out=w1639:refnum<vi>, error out=w1644:errorcluster, "Value"=w1643:string)  [unwired: 1 in]
                n684 = Concatenate Strings(w1643, "Done!" ("string")) -> (w1642:string)
                n685 = Enqueue Element At Opposite End(queue=w1648, element="unzip", error in (no error)=w1645) -> (error out=w1647:errorcluster)  [unwired: 1 in, 2 out]
                n686 = property class="Str"(reference=w1639, error in=w1644, "Value"=w1642) -> ()  [unwired: 2 out]
              }
              frame Error {
                n687 = Bundle By Name(cluster=w1650, "Error"="Error al ejecutar el cmd shell", "Pass?"="False") -> (w1649:T2)
              }
            }
          }
          frame "unzip" {
            n688 = Unbundle By Name(w1666) -> ("Media version"=w1665:i32, "My temp"=w1657:path)
            n689 = Number To Decimal String(number=w1665) -> (decimal integer string=w1669:string)  [unwired: 1 in]
            n690 = Concatenate Strings(w1669, ".zip" ("string")) -> (w1670:string)
            n691 = String To Path(string=w1670) -> (path=w1667:path)
            n692 = Build Path(base path=path "C:/GUIMedia", name or relative path=w1667) -> (appended path=w1658:path)
            n693 = call <vilib>:"Check if File or Folder Exists.vi"("path"=w1657) -> ("error out"=w1660:errorcluster, "file or folder exists?"=w1661:bool, "dup path"=w1656:path)  [unwired: 8 in]
            n694 = case shown="True" w1661 {
              tunnel: [w1673 w1679] -> _
              tunnel: [w1672 w1678] -> w1659
              tunnel: w1660 -> [w1674 w1680]
              tunnel: w1656 -> [_ w1675]
              frame False {
                n695 = Create Folder(error in=w1674) -> (created path=w1673:path, error out=w1672:errorcluster)  [unwired: 2 in, 1 out]
              }
              frame True {
                n696 = Delete(path (use dialog)=w1675, entire hierarchy (F)=TRUE, error in=w1680) -> (deleted path=w1677:path, error out=w1676:errorcluster)  [unwired: 2 in, 1 out]
                n697 = Create Folder(path (use dialog)=w1677, error in=w1676) -> (created path=w1679:path, error out=w1678:errorcluster)  [unwired: 1 in, 1 out]
              }
            }
            n698 = call <vilib>:"Unzip.vi"("error in (no error)"=w1659, "Target directory (same as Zip file if empty)"=w1657, "Zip file"=w1658) -> ()  [unwired: 6 in, 3 out]
            n699 = Enqueue Element(queue=w1655, element="send files", error in (no error)=w1654) -> (error out=w1664:errorcluster)  [unwired: 1 in, 2 out]
          }
          frame "send files" {
            w1697 = "\"" ("input 1")
            n700 = Unbundle By Name(w1685) -> ("Console"=w1704:refnum<vi>, "Version path"=w1692:path, "My temp"=w1691:path)
            n701 = property class="Str"(reference=w1704) -> (reference out=w1705:refnum<vi>, "Value"=w1703:string)  [unwired: 1 in, 1 out]
            n702 = call "Progress bar.vi"("TIme (s)"=130.0, "Title"="Sending media") -> ()  [unwired: 9 in, 1 out]
            n703 = property on="Status" class="Str"("Value"="Actualizando archivos multimedia" ("Status"), "Text.FontSize"=u32 32 ("Text.Font:Size")) -> ()  [unwired: 2 in, 2 out]
            n704 = Concatenate Strings(w1703, "\nSending files...\n" ("string")) -> (w1702:string)
            n705 = Path To String(path=w1691) -> (string=w1698:string)
            n706 = property class="Str"(reference=w1705, "Value"=w1702) -> (reference out=w1701:refnum<vi>)  [unwired: 1 in, 1 out]
            n707 = Concatenate Strings("adb push " ("initial string"), w1697, w1698, w1697, " /sdcard/media/" ("input 2")) -> (w1695:string)
            n708 = call <vilib>:"System Exec.vi"("run minimized? (F)"=TRUE, "working directory"=w1692, "command line"=w1695) -> ("error out"=w1687:errorcluster, "standard error"=w1707:string, "standard output"=w1686:string)  [unwired: 5 in, 1 out]
            n709 = property class="Str"(reference=w1701) -> (reference out=w1714:refnum<vi>, error out=w1711:errorcluster, "Value"=w1713:string)  [unwired: 1 in]
            n710 = Concatenate Strings(w1713, w1686, w1707) -> (w1712:string)
            n711 = property class="Str"(reference=w1714, error in=w1711, "Value"=w1712) -> ()  [unwired: 2 out]
            n712 = Match Pattern(string=w1686, regular expression="adb: error") -> (offset past match=w1689:i32)  [unwired: 1 in, 3 out]
            n713 = Greater Or Equal To 0?(x=w1689) -> (x >= 0?=w1688:bool)
            n714 = case shown="True" w1688 {
              tunnel: w1710 -> [w1720 w1727]
              tunnel: [w1719 w1728] -> w1706
              tunnel: w1687 -> [w1716 w1729]
              tunnel: w1685 -> [w1715 w1725]
              tunnel: [w1715 w1726] -> w1684
              frame False {
                n715 = call <vilib>:"Close Progress Bar.vi"() -> ("error out"=w1717:errorcluster)  [unwired: 10 in, 1 out]
                n716 = call <vilib>:"Clear Errors.vi"("error in (no error)"=w1717) -> ()  [unwired: 5 in, 2 out]
                n717 = Enqueue Element At Opposite End(queue=w1720, element="mv temp -> media", error in (no error)=w1716) -> (error out=w1719:errorcluster)  [unwired: 1 in, 2 out]
              }
              frame True {
                n718 = Unbundle By Name(w1725) -> ("Attempts left"=w1723:i32)
                n719 = call <vilib>:"Close Progress Bar.vi"() -> ("error out"=w1730:errorcluster)  [unwired: 10 in, 1 out]
                n720 = call <vilib>:"Clear Errors.vi"("error in (no error)"=w1730) -> ()  [unwired: 5 in, 2 out]
                n721 = Less Or Equal To 0?(x=w1723) -> (x <= 0?=w1722:bool)
                n722 = case shown="False" w1722 {
                  tunnel: w1729 -> [w1734 w1740]
                  tunnel: [w1733 w1739] -> w1728
                  tunnel: w1727 -> [w1732 w1738]
                  tunnel: "Ocurrió un problema y en algún momento\nse perdió la conexión con el GUI" -> [_ w1736]
                  frame False {
                    n723 = Enqueue Element At Opposite End(queue=w1732, element="update media", error in (no error)=w1734) -> (error out=w1733:errorcluster)  [unwired: 1 in, 2 out]
                  }
                  frame True {
                    n724 = call "Custom User Message.vi"("Button text (\"OK\")"="OK" ("Button text (\"OK\")"), "MSG"=w1736) -> ()  [unwired: 9 in, 1 out]
                    n725 = Enqueue Element At Opposite End(queue=w1738, element="error", error in (no error)=w1740) -> (error out=w1739:errorcluster)  [unwired: 1 in, 2 out]
                  }
                }
                n726 = Decrement(x=w1723) -> (x-1=w1724:i32)
                n727 = Bundle By Name(cluster=w1725, "Attempts left"=w1724) -> (w1726:T2)
              }
            }
          }
          frame "mv temp -> media" {
            n728 = Unbundle By Name(w1752) -> ("Console"=w1755:refnum<vi>, "Version path"=w1741:path, "Media version"=w1748:i32)
            n729 = Format Into String(format string="adb shell mv /sdcard/media/temp /sdcard/media/%d" ("command line"), w1748) -> (resulting string=w1745:string)  [unwired: 2 in, 1 out]
            n730 = property class="Str"(reference=w1755) -> (reference out=w1756:refnum<vi>, "Value"=w1754:string)  [unwired: 1 in, 1 out]
            n731 = Concatenate Strings(w1754, "\r", ">" ("string"), w1745) -> (w1753:string)
            n732 = property class="Str"(reference=w1756, "Value"=w1753) -> (reference out=w1744:refnum<vi>)  [unwired: 1 in, 1 out]
            n733 = property class="Str"(reference=w1744, "Text.Scroll Position"=u32 4294967295) -> (reference out=w1742:refnum<vi>)  [unwired: 1 in, 1 out]
            n734 = call <vilib>:"System Exec.vi"("run minimized? (F)"=TRUE, "working directory"=w1741, "command line"=w1745) -> ("error out"=w1751:errorcluster, "standard error"=w1758:string, "standard output"=w1762:string)  [unwired: 5 in, 1 out]
            n735 = property class="Str"(reference=w1742) -> (reference out=w1766:refnum<vi>, error out=w1763:errorcluster, "Value"=w1765:string)  [unwired: 1 in]
            n736 = Concatenate Strings(w1765, w1762, w1758) -> (w1764:string)
            n737 = property class="Str"(reference=w1766, error in=w1763, "Value"=w1764) -> (reference out=w1750:refnum<vi>)  [unwired: 1 out]
            n738 = case shown="No Error" w1751 {
              selector: w1751 -> [w1767 w1771]
              tunnel: w1761 -> [w1770 _]
              tunnel: [w1769 w1771] -> w1757
              tunnel: w1750 -> [_ _]
              frame No Error {
                n739 = Enqueue Element At Opposite End(queue=w1770, element="end", error in (no error)=w1767) -> (error out=w1769:errorcluster)  [unwired: 1 in, 2 out]
              }
              frame Error {
              }
            }
          }
          frame "end" {
            n740 = Unbundle By Name(w1777) -> ("ID Part"=w1775:string, "IO task"=w1773:refnum<k24>)
            n741 = flat-sequence {
              frame #0 {
                n742 = call "Custom User Message.vi"("Button text (\"OK\")"="OK" ("Button text (\"OK\")"), "MSG"="\n\n¡Passed/Paso!\n" ("message")) -> ()  [unwired: 9 in, 1 out]
              }
              frame #1 {
                n743 = property on="Stop button" class="Bool (strict)"("Val(Sgnl)"=TRUE ("Value (Signaling)")) -> ()  [unwired: 2 in, 2 out]
                n744 = property on="Status" class="Str"("Visible"=TRUE, "Text.TextColors"=T9 {"Text Color"=16777228, "Background Color"=6618880} ("Text.Text Colors"), "Value"="PASSED!" ("Status"), "Text.FontSize"=u32 71 ("Text.Font:Size")) -> ()  [unwired: 2 in, 2 out]
              }
            }
            n745 = call-poly <vilib>:"ULx Write.vi"("task in"=w1773, "data"=FALSE) -> ("error out"=w1772:errorcluster)  [unwired: 11 in, 2 out]
            n746 = call "Log File Results.vi"("Error"="", "Pass?"="True", "Part Number"=w1775) -> ()  [unwired: 8 in, 1 out]
          }
          frame "kill loop" {
          }
          frame "legacy install media" {
            n747 = Unbundle By Name(w1799) -> ("Console"=w1795:refnum<vi>, "Python session"=w1803:refnum<k35>, "Script path"=w1802:path, "Media version"=w1790:i32)
            n748 = property class="Str"(reference=w1795) -> (reference out=w1808:refnum<vi>, error out=w1805:errorcluster, "Value"=w1807:string)  [unwired: 1 in]
            n749 = Concatenate Strings(w1807, "\n>Installing media...\n" ("function name")) -> (w1806:string)
            n750 = property class="Str"(reference=w1808, error in=w1805, "Value"=w1806) -> (reference out=w1793:refnum<vi>, error out=w1791:errorcluster)
            n751 = node(w1803, w1802, "install_media" ("function name"), w1791, w1790, w1790) -> (w1797:refnum<k35>, w1798:errorcluster)  [unwired: 2 in, 2 out]
            n752 = Close Python Session(session in=w1797, error in=w1798) -> (11:w1796:errorcluster)
            n753 = case shown="No Error" w1796 {
              selector: w1796 -> [w1809 w1819]
              tunnel: w1800 -> [w1818 w1821]
              tunnel: [w1816 w1822] -> w1801
              tunnel: w1793 -> [w1810 _]
              frame No Error {
                n754 = disable-structure shown="Disabled" {
                  frame Disabled {
                    n755 = call <vilib>:"Close Progress Bar.vi"() -> ()  [unwired: 10 in, 2 out]
                  }
                  frame Enabled {
                  }
                }
                n756 = property class="Str"(reference=w1810) -> (reference out=w1815:refnum<vi>, error out=w1814:errorcluster, "Value"=w1813:string)  [unwired: 1 in]
                n757 = Concatenate Strings(w1813, "Done!" ("string")) -> (w1812:string)
                n758 = property class="Str"(reference=w1815, error in=w1814, "Value"=w1812) -> ()  [unwired: 2 out]
                n759 = Enqueue Element(queue=w1818, element="end", error in (no error)=w1809) -> (error out=w1816:errorcluster)  [unwired: 1 in, 2 out]
              }
              frame Error {
                n760 = disable-structure shown="Disabled" {
                  frame Disabled {
                    n761 = call <vilib>:"Close Progress Bar.vi"() -> ()  [unwired: 10 in, 2 out]
                  }
                  frame Enabled {
                  }
                }
                n762 = Enqueue Element(queue=w1821, element="error", error in (no error)=w1819) -> (error out=w1822:errorcluster)  [unwired: 1 in, 2 out]
              }
            }
          }
        }
      }
      frame Error {
        n763 = call <vilib>:"Simple Error Handler.vi"("error in (no error)"=w1835) -> ("code out"=w1840:i32, "error out"=w1839:errorcluster)  [unwired: 4 in, 3 out]
        n764 = Unbundle By Name(w1842) -> ("Error"=w1830:string, "ID Part"=w1833:string, "Pass?"=w1831:string, "COM"=w1841:refnum<visa-resource-name>, "IO task"=w1825:refnum<k24>)
        n765 = call <vilib>:"Clear Errors.vi"("error in (no error)"=w1839, "specific error code to clear (0: all)"=w1840) -> ("error out"=w1836:errorcluster)  [unwired: 4 in, 1 out]
        n766 = Flush Queue(queue=w1843, error in (no error)=w1836) -> (error out=w1828:errorcluster)  [unwired: 2 out]
        n767 = Equal?(x=w1831, y="False") -> (x = y?=w1834:bool)
        n768 = VISA Close(VISA resource name=w1841, error in (no error)=w1835) -> (error out=w1837:errorcluster)
        n769 = call-poly <vilib>:"ULx Write.vi"("task in"=w1825, "data"=FALSE) -> ("error out"=w1824:errorcluster)  [unwired: 11 in, 2 out]
        n770 = call <vilib>:"Clear Errors.vi"("error in (no error)"=w1837) -> ()  [unwired: 5 in, 2 out]
        n771 = call <vilib>:"Clear Errors.vi"("error in (no error)"=w1824) -> ("error out"=w1823:errorcluster)  [unwired: 5 in, 1 out]
        n772 = case shown="True" w1834 {
          tunnel: w1833 -> [_ w1854]
          tunnel: w1831 -> [_ w1853]
          tunnel: w1830 -> [_ w1852]
          tunnel: [_ w1848] -> w1829
          frame False {
          }
          frame True {
            n773 = call "Log File Results.vi"("Error"=w1852, "Pass?"=w1853, "Part Number"=w1854) -> ("error out"=w1847:errorcluster)  [unwired: 8 in]
            n774 = property on="Status" class="Str"(error in=w1847, "Visible"=TRUE, "Text.TextColors"=T9 {"Text Color"=16777225, "Background Color"=16711680} ("Text.Text Colors"), "Value"="FAILED!" ("Status"), "Text.FontSize"=u32 71 ("Text.Font:Size")) -> (error out=w1848:errorcluster)  [unwired: 1 in, 1 out]
          }
        }
        n775 = Merge Errors(w1829, w1823, w1828) -> (w1827:errorcluster)
        n776 = property on="Stop button" class="Bool (strict)"(error in=w1827, "Val(Sgnl)"=TRUE ("Value (Signaling)")) -> (error out=w1838:errorcluster)  [unwired: 1 in, 1 out]
      }
    }
  }
  n777 = while {
    shift-right: [w1860] -> w54
    shift-left: w31 -> [w1861]
    tunnel: w52 -> [w1862]
    tunnel: [w1858] -> w11
    tunnel: w5 -> [w1857]
    tunnel: w14 -> [w1856]
    stop <- w1855 stop-if-true
    # "This loop is the producer loop."
    # "Event handler"
    n778 = event shown="[6] <stop app>: User Event" {
      selector: w1856 -> [_ _ _ _ _ _ _]
      dyn-events: [_ _ _ _ _ _ _] -> w1858
      timeout: _ -> [_ _ _ _ _ _ _]
      tunnel: w1862 -> [w1866 w1879 w1890 w1903 w1909 w1919 _]
      tunnel: w1861 -> [w1865 w1878 w1891 w1904 w1910 w1916 w1921]
      tunnel: [w1864 w1877 w1888 w1902 w1912 w1915 _] -> w1860
      tunnel: [_ _ _ _ _ _ TRUE] -> w1859
      tunnel: w1857 -> [_ _ _ w1905 w1908 _ w1922]
      event "Settings button": Value Change {
        n779 = event-data() -> ("NewVal"=w1863:bool)  [unwired: 1 in]
        n780 = case shown="False" w1863 {
          tunnel: w1866 -> [w1869 w1875]
          tunnel: w1865 -> [w1871 w1874]
          tunnel: [w1868 w1873] -> w1864
          frame False {
            n781 = Enqueue Element(queue=w1869, element="close settings", error in (no error)=w1871) -> (error out=w1868:errorcluster)  [unwired: 1 in, 2 out]
            n782 = property on="Paths" class="Bool (strict)"("Val(Sgnl)"=FALSE ("Value (Signaling)")) -> ()  [unwired: 2 in, 2 out]
          }
          frame True {
            n783 = Enqueue Element(queue=w1875, element="open settings", error in (no error)=w1874) -> (error out=w1873:errorcluster)  [unwired: 1 in, 2 out]
          }
        }
      }
      event "Paths": Value Change {
        n784 = event-data() -> ("NewVal"=w1876:bool)  [unwired: 1 in]
        n785 = case shown="True" w1876 {
          tunnel: w1879 -> [w1880 w1887]
          tunnel: w1878 -> [w1882 w1886]
          tunnel: [w1883 w1885] -> w1877
          frame False {
            n786 = Enqueue Element(queue=w1880, element="close paths", error in (no error)=w1882) -> (error out=w1883:errorcluster)  [unwired: 1 in, 2 out]
          }
          frame True {
            n787 = Enqueue Element(queue=w1887, element="open paths", error in (no error)=w1886) -> (error out=w1885:errorcluster)  [unwired: 1 in, 2 out]
          }
        }
      }
      event "Save button": Value Change {
        n788 = event-data() -> ("NewVal"=w1889:bool)  [unwired: 1 in, 2 out]
        n789 = case shown="True" w1889 {
          tunnel: w1890 -> [_ w1896]
          tunnel: w1891 -> [w1892 w1895]
          tunnel: [w1892 w1894] -> w1888
          frame False {
          }
          frame True {
            n790 = Enqueue Element(queue=w1896, element="save config", error in (no error)=w1895) -> (error out=w1894:errorcluster)  [unwired: 1 in, 2 out]
          }
        }
      }
      event "Run button": Value Change {
        n791 = event-data() -> ("NewVal"=w1897:bool)  [unwired: 1 in, 5 out]
        n792 = case shown="True" w1897 {
          frame False {
          }
          frame True {
            n793 = property on="Settings button" class="Bool (strict)"("Val(Sgnl)"=FALSE ("Value (Signaling)")) -> ()  [unwired: 2 in, 2 out]
          }
        }
        n794 = Enqueue Element(queue=w1903, element="running") -> (error out=w1900:errorcluster)  [unwired: 2 in, 2 out]
        n795 = Enqueue Element(queue=w1905, element="validate config", error in (no error)=w1904) -> (error out=w1901:errorcluster)  [unwired: 1 in, 2 out]
        n796 = Merge Errors(w1900, w1901) -> (w1902:errorcluster)
      }
      event "Stop button": Value Change {
        n797 = event-data() -> ()  [unwired: 1 in, 6 out]
        n798 = Enqueue Element At Opposite End(queue=w1909, element="idle", error in (no error)=w1910) -> (error out=w1914:errorcluster)  [unwired: 1 in, 2 out]
        n799 = Enqueue Element At Opposite End(queue=w1908, element="idle", error in (no error)=w1910) -> (error out=w1907:errorcluster)  [unwired: 1 in, 2 out]
        n800 = Merge Errors(w1914, w1907) -> (w1912:errorcluster)
      }
      event Panel Close? {
        n801 = event-data() -> ()  [unwired: 1 in, 3 out]
        n802 = Enqueue Element At Opposite End(queue=w1919, element="confirm quit", error in (no error)=w1916) -> (error out=w1915:errorcluster)  [unwired: 1 in, 2 out]
        n803 = event-data("Discard?"=TRUE) -> ()  [unwired: 1 in, 1 out]
      }
      event User Event {
        n804 = event-data() -> ()  [unwired: 1 in, 3 out]
        n805 = Enqueue Element At Opposite End(queue=w1922, element="kill loop", error in (no error)=w1921) -> ()  [unwired: 1 in, 3 out]
      }
    }
    n806 = Or(x=w1860, y=w1859) -> (x .or. y?=w1855:bool)
  }
  n807 = control-ref of="Paths"() -> (w21:refnum<vi>)
  n808 = Bundle("secondary color"=w18, "secondary color"=w18) -> (w17:T14)  [unwired: 1 in]
  n809 = call "button painter (SubVI).vi"("Off state"=w17, "On state"=w20, "Button ref in"=w21) -> ()  [unwired: 9 in]
  n810 = while {
    tunnel: w52 -> [w1932]
    shift-right: [w1927] -> _
    shift-left: w50 -> [w1928]
    tunnel: w44 -> [w1925]
    tunnel: [w1924] -> w7
    stop <- w1930 stop-if-true
    # "This loop is a consumer loop."
    # "UI consummer"
    n811 = Dequeue Element(queue=w1932) -> (queue out=w1926:refnum<queue>, element=w1929:string, error out=w1931:errorcluster)  [unwired: 2 in, 1 out]
    n812 = case shown="Error" w1931 {
      tunnel: [_ TRUE] -> w1930
      tunnel: w1929 -> [w1938 _]
      tunnel: w1928 -> [w1937 _]
      tunnel: [w1936 _] -> w1927
      tunnel: w1926 -> [w1935 _]
      tunnel: w1925 -> [w1934 _]
      tunnel: [w1933 _] -> w1924
      frame No Error {
        # "Process the data here."
        n813 = case shown="\"exit\"" w1938 {
          tunnel: w1937 -> [w1950 w1962 w1967 w1976 w1997 w2016 w2024 w2036 w2044 w2052 w2061]
          tunnel: [w1949 w1962 w1967 w1976 w1997 w2016 w2024 w2036 w2044 w2052 w2061] -> w1936
          tunnel: w1935 -> [w1947 _ _ _ _ _ _ _ _ w2051 _]
          tunnel: w1934 -> [_ _ _ _ _ _ _ _ _ _ w2060]
          tunnel: [w1939 _ _ w1968 w1982 w2014 w2022 w2030 w2038 w2046 w2056] -> w1933
          frame "init", Default {
            n814 = Enqueue Element(queue=w1947, element="read config") -> (queue out=w1943:refnum<queue>, error out=w1945:errorcluster)  [unwired: 2 in, 1 out]
            n815 = Enqueue Element(queue=w1943, element="idle", error in (no error)=w1945) -> (error out=w1939:errorcluster)  [unwired: 1 in, 2 out]
            n816 = control-ref of="footer splitter"() -> (w1948:refnum<vi>)
            n817 = control-ref of="Serial communication\n settings"() -> (w1940:refnum<vi>)
            n818 = control-ref of="Path: Android OS"() -> (w1942:refnum<vi>)
            n819 = control-ref of="Path: 4.9.12.XXXX"() -> (w1941:refnum<vi>)
            n820 = control-ref of="settings splitter"() -> (w1951:refnum<vi>)
            n821 = Bundle By Name(cluster=w1950, "settings splitter"=w1951, "footer splitter"=w1948, "Serial communication\n settings"=w1940, "Path: Android OS"=w1942, "Path: 4.9.12.XXXX"=w1941) -> (w1949:T4)
          }
          frame "idle" {
            n822 = property on="Save button" class="Bool (strict)"("DisabledEnum"=T3."Enabled" ("Disabled"), "Value"=FALSE ("Save button")) -> ()  [unwired: 2 in, 2 out]
            n823 = property on="Settings button" class="Bool (strict)"("DisabledEnum"=T3."Enabled" ("Disabled"), "Val(Sgnl)"=FALSE ("Settings")) -> ()  [unwired: 2 in, 2 out]
            n824 = property on="Run button" class="Bool (strict)"("DisabledEnum"=T3."Enabled" ("Disabled"), "Value"=FALSE ("Save button")) -> ()  [unwired: 2 in, 2 out]
            n825 = property on="Stop button" class="Bool (strict)"("DisabledEnum"=T3."Disabled" ("Disabled"), "Value"=FALSE ("Save button")) -> ()  [unwired: 2 in, 2 out]
            n826 = property on="Paths" class="Bool (strict)"("DisabledEnum"=T3."Enabled" ("Disabled"), "Val(Sgnl)"=FALSE ("Paths")) -> ()  [unwired: 2 in, 2 out]
          }
          frame "running" {
            n827 = property on="Run button" class="Bool (strict)"("DisabledEnum"=T3."Disabled" ("Disabled")) -> ()  [unwired: 2 in, 2 out]
            n828 = property on="Stop button" class="Bool (strict)"("Value"=TRUE ("Stop button"), "DisabledEnum"=T3."Enabled" ("Disabled")) -> ()  [unwired: 2 in, 2 out]
            n829 = property on="Settings button" class="Bool (strict)"("DisabledEnum"=T3."Disabled and Grayed Out" ("Disabled")) -> ()  [unwired: 2 in, 2 out]
          }
          frame "read config" {
            n830 = Unbundle By Name(w1976) -> ("Path: Android OS"=w1972:refnum<vi>, "Path: 4.9.12.XXXX"=w1975:refnum<vi>, "Serial communication\n settings"=w1970:refnum<vi>)
            n831 = call "settings handler.vi"("Operation"=enum16{"Open", "Write", "Read", "Close"}."Open") -> ("Error Out"=w1979:errorcluster)  [unwired: 8 in, 2 out]
            n832 = call "settings handler.vi"("Operation"=enum16{"Open", "Write", "Read", "Close"}."Read", "error in (no error)"=w1979) -> ("Paths read"=w1974:T11, "Read"=w1969:T1)  [unwired: 7 in, 1 out]
            n833 = property class="Clust (strict)"(reference=w1970, "Value"=w1969) -> ()  [unwired: 1 in, 2 out]
            n834 = Unbundle By Name(w1974) -> ("Version"=w1973:path, "Android"=w1971:path)
            n835 = property class="Path"(reference=w1975, "Value"=w1973) -> ()  [unwired: 1 in, 2 out]
            n836 = property class="Path"(reference=w1972, "Value"=w1971) -> (error out=w1968:errorcluster)  [unwired: 1 in, 1 out]
          }
          frame "save config" {
            n837 = Unbundle By Name(w1997) -> ("Serial communication\n settings"=w1996:refnum<vi>, "Path: Android OS"=w1995:refnum<vi>, "Path: 4.9.12.XXXX"=w1994:refnum<vi>)
            n838 = property on="Save button" class="Bool (strict)"("DisabledEnum"=T3."Disabled and Grayed Out" ("Disabled")) -> ()  [unwired: 2 in, 2 out]
            n839 = property class="Path"(reference=w1994) -> ("Value"=w1992:path)  [unwired: 1 in, 2 out]
            n840 = property class="Clust (strict)"(reference=w1996) -> ("Value"=w1987:T1)  [unwired: 1 in, 2 out]
            n841 = property class="Path"(reference=w1995) -> ("Value"=w1993:path)  [unwired: 1 in, 2 out]
            n842 = Unbundle By Name(w1987) -> ("Board IP"=w1986:string)
            n843 = Bundle("Value"=w1993, "Value"=w1992, path "", path "", path "") -> (w1991:T15)  [unwired: 1 in]
            n844 = call "IP check.vi"("IP address string"=w1986) -> ("Valid?"=w1985:bool)  [unwired: 10 in]
            n845 = case shown="True" w1985 {
              tunnel: w1991 -> [_ w2004]
              tunnel: w1987 -> [_ w2002]
              tunnel: [_ w2000] -> w1983
              frame False {
                n846 = call "Custom User Message.vi"("Button text (\"OK\")"="OK" ("Button text (\"OK\")"), "MSG"="\nError al guardar: \n-IP invalida.\n") -> ()  [unwired: 9 in, 1 out]
              }
              frame True {
                n847 = call "settings handler.vi"("Operation"=enum16{"Open", "Write", "Read", "Close"}."Write", "Paths write"=w2004, "Write"=w2002) -> ("Error Out"=w2003:errorcluster)  [unwired: 6 in, 2 out]
                n848 = case shown="Error .." w2003 {
                  selector: w2003 -> [w2010 _]
                  tunnel: [w2005 _] -> w2000
                  frame No Error {
                    n849 = call "settings handler.vi"("Operation"=enum16{"Open", "Write", "Read", "Close"}."Close", "error in (no error)"=w2010) -> ("Error Out"=w2008:errorcluster)  [unwired: 7 in, 2 out]
                    n850 = call "Custom User Message.vi"("Button text (\"OK\")"="OK" ("Button text (\"OK\")"), "MSG"="\n\n¡Se ha guardado con éxito!") -> ()  [unwired: 9 in, 1 out]
                    n851 = call "settings handler.vi"("Operation"=enum16{"Open", "Write", "Read", "Close"}."Open", "error in (no error)"=w2008) -> ("Error Out"=w2005:errorcluster)  [unwired: 7 in, 2 out]
                  }
                  frame Error {
                    n852 = call "Custom User Message.vi"("Button text (\"OK\")"="OK" ("Button text (\"OK\")"), "MSG"="\n\n¡Se ha producido un error al guardar!") -> ()  [unwired: 9 in, 1 out]
                  }
                }
              }
            }
            n853 = property on="Save button" class="Bool (strict)"(error in=w1983, "Value"=FALSE ("Save button"), "DisabledEnum"=T3."Enabled" ("Disabled")) -> (error out=w1982:errorcluster)  [unwired: 1 in, 1 out]
          }
          frame "open settings" {
            n854 = Unbundle By Name(w2016) -> ("settings splitter"=w2018:refnum<vi>, "footer splitter"=w2017:refnum<vi>)
            n855 = property class="Splitter"(reference=w2017) -> (error out=w2015:errorcluster, "Width"=w2021:u32)  [unwired: 1 in, 1 out]
            n856 = Subtract(x=w2021, y=u32 240) -> (x-y=w2020:u32)
            n857 = property class="Splitter"(reference=w2018, error in=w2015, "Position"=w2020) -> (error out=w2014:errorcluster)  [unwired: 1 out]
          }
          frame "close settings" {
            n858 = Unbundle By Name(w2024) -> ("settings splitter"=w2026:refnum<vi>, "footer splitter"=w2025:refnum<vi>)
            n859 = property class="Splitter"(reference=w2025) -> (error out=w2023:errorcluster, "Width"=w2029:u32)  [unwired: 1 in, 1 out]
            n860 = Subtract(x=w2029, y=u32 6) -> (x-y=w2028:u32)
            n861 = property class="Splitter"(reference=w2026, error in=w2023, "Position"=w2028) -> (error out=w2022:errorcluster)  [unwired: 1 out]
          }
          frame "open paths" {
            n862 = control-ref of="This VI"() -> (w2035:refnum<vi>)
            n863 = Unbundle By Name(w2036) -> ("footer splitter"=w2037:refnum<vi>)
            n864 = property class="VI"(reference=w2035) -> ("Panel"=w2034:refnum<vi>)  [unwired: 1 in, 2 out]
            n865 = property class="Pnl"(reference=w2034) -> ("Height"=w2033:u32)  [unwired: 1 in, 2 out]
            n866 = Subtract(x=w2033, y=u32 125) -> (x-y=w2031:u32)
            n867 = property class="Splitter"(reference=w2037, "Position"=w2031) -> (error out=w2030:errorcluster)  [unwired: 1 in, 1 out]
          }
          frame "close paths" {
            n868 = control-ref of="This VI"() -> (w2043:refnum<vi>)
            n869 = Unbundle By Name(w2044) -> ("footer splitter"=w2045:refnum<vi>)
            n870 = property class="VI"(reference=w2043) -> ("Panel"=w2042:refnum<vi>)  [unwired: 1 in, 2 out]
            n871 = property class="Pnl"(reference=w2042) -> ("Height"=w2041:u32)  [unwired: 1 in, 2 out]
            n872 = Subtract(x=w2041, y=u32 28) -> (x-y=w2040:u32)
            n873 = property class="Splitter"(reference=w2045, "Position"=w2040) -> (error out=w2038:errorcluster)  [unwired: 1 in, 1 out]
          }
          frame "confirm quit" {
            n874 = call "Two BTN Custom User Message.vi"("Option 2 (\"Stop\")"="Cancelar" ("F button name (\"Cancel\")"), "Option 1 (\"OK\")"="Si" ("T button name (\"OK\")"), "Message"="\n\n¿Seguro que quiere cerrar\nla aplicación?" ("message")) -> ("Ok?"=w2049:bool)  [unwired: 8 in]
            n875 = case shown="True" w2049 {
              tunnel: w2051 -> [_ w2055]
              tunnel: [_ w2053] -> w2046
              frame False {
              }
              frame True {
                n876 = Enqueue Element At Opposite End(queue=w2055, element="exit" ("Message")) -> (error out=w2053:errorcluster)  [unwired: 2 in, 2 out]
              }
            }
          }
          frame "exit" {
            n877 = call "settings handler.vi"("Operation"=enum16{"Open", "Write", "Read", "Close"}."Close") -> ("Error Out"=w2058:errorcluster)  [unwired: 8 in, 2 out]
            n878 = Generate User Event(user event=w2060, event data cluster="stop app" ("event data"), error in=w2058) -> (error out=w2056:errorcluster)  [unwired: 1 in, 1 out]
          }
        }
      }
      frame Error {
        # "Return true in any case that should stop the loop."
        n879 = disable-structure "Conditional Disable Structure" shown="RUN_TIME_ENGINE==True&&OS==Win" {
          frame condition #0 (active) {
          }
          frame condition #1 {
            n880 = Quit LabVIEW(quit? (T)=TRUE) -> ()
          }
        }
      }
    }
  }
  n881 = Release Queue(queue=w52, error in (no error)=w54) -> (error out=w10:errorcluster)  [unwired: 1 in, 2 out]
  n882 = Merge Errors(w7, w10, w8) -> (w9:errorcluster)
  n883 = Release Queue(queue=w5, error in (no error)=w9) -> (error out=w6:errorcluster)  [unwired: 1 in, 2 out]
  n884 = Unregister For Events(event registration refnum=w11, error in=w6) -> ()  [unwired: 1 out]
